vi "Control Experiment.vi"(8 "Error In":errorcluster, 9 "KH":T5={"KH #"=[0, 1, 2, 3, 4, 5, 6, 7, 8, 9, 10, 11, 12, 13, 14, 15], "KH Configuration"=[enum."SE+ (-gnd)", enum."SE+ (-gnd)", enum."Differential", enum."Differential", enum."SE+ (-gnd)", enum."Differential", enum."Differential", enum."SE+ (-gnd)", enum."Differential", enum."Differential", enum."SE+ (-gnd)", enum."SE+ (-gnd)", enum."Differential", enum."Ground", enum."Ground", enum."Ground"], "KH Gain"=[enum."1000x", enum."1000x", enum."1000x", enum."1000x", enum."1000x", enum."1000x", enum."1000x", enum."1000x", enum."1000x", enum."1000x", enum."1000x", enum."1000x", enum."1000x", enum."1000x", enum."1000x", enum."100x"], "KH Shunt Resistor"=[enum."Open", enum."Open", enum."Open", enum."5k Ohms", enum."Open", enum."Open", enum."5k Ohms", enum."Open", enum."Open", enum."5k Ohms", enum."Open", enum."Open", enum."50k Ohms", enum."Open", enum."Open", enum."Open"]}, 10 "Lockin":T7={"AI"=[1, 2, 3, 4, 5, 6, 7, 8, 9, 10, 11, 12, 13, 14, 15, 16], "Electrode"=["4", "5", "6", "7", "9", "11", "12", "13", "16", "17", "20", "21", "1", "", "", ""], "Label"=[12, 14, 15, 13, 10, 11, 9, 8, 4, 2, 1, 3, 6, 0, 0, 0], "Electrode Config"=[enum."Current", enum."Voltage (SE)", enum."Voltage (SE)", enum."Current", enum."Voltage (SE)", enum."Voltage (SE)", enum."Current", enum."Current", enum."Voltage (SE)", enum."Current", enum."Current", enum."Voltage (SE)", enum."Gate", enum."Voltage (SE)", enum."Voltage (SE)", enum."Voltage (SE)"]} {"Label" items=["", "I+", "I-", "V1+", "V1-", "dV1", "Vsg", "Vbg", "I2+", "I2-", "V2+", "V2-", "I3+", "I3-", "V3+", "V3-"]}) -> (0 "Error Out":errorcluster)   [LabVIEW 2019, in "Control Experiment.lvclass"]
doc: "Use this VI to help configure your experiment.\n1. Choose Pickering or Not Pickering\n2. Configure the Electrode control to show which electrode is connected to which lockin\n3. Choose a Label for each electrode to configure Krohn Hite amplifier automatically\n4. Easily set all Krohn Hite channels to be \"all ground\" or \"all differential\" mode\n5. Fill out information about you and your device in the lower left corner\n6. When you are finished, or when you want to update the amplifiers, click the \"CREATE OUTPUT\" button located in upper right. Clicking this button will set the amplifiers, Pickering switch (if you have one), and write information to a functional global variable that you can easily read from elsewhere in your program"
uses:
  Control Experiment.lvclass
  Typedefs/Instrument--enum.ctl
  <userlib>/LevyLab/Krohn Hite 7008/typedefs/Shunt-Enum.ctl
  Typedefs/KH Mode-enum.ctl
  <userlib>/LevyLab/Krohn Hite 7008/typedefs/Input Configuration-Enum.ctl
  <userlib>/LevyLab/Krohn Hite 7008/typedefs/Gain-Enum.ctl
  <userlib>/LevyLab/Krohn Hite 7008/typedefs/SetAll-Array.ctl
  <userlib>/LevyLab/Krohn Hite 7008/typedefs/SetAll-Cluster.ctl
  <userlib>/LevyLab/Krohn Hite 7008/typedefs/Channel-Enum.ctl
  <userlib>/LevyLab/Krohn Hite 7008/typedefs/Filter-Enum.ctl
  <userlib>/LevyLab/Krohn Hite 7008/typedefs/Coupling-Enum.ctl
  <userlib>/LevyLab/Instrument Framework/SMOs/Configuration/Configuration.lvclass
  Typedefs/UI Controls --cluster.ctl
  <userlib>/LevyLab/Instrument Framework/SMOs/Logger.PGSQL/Logger.PGSQL.lvclass
  C:/Program Files (x86)/National Instruments/LabVIEW 2019/vi.lib/JKI/JKI SMO/SMO/SMO.lvclass
  Control Experiment.lvclass/Control Experiment.ctl
  <userlib>/_MGI/File/MGI Create Directory Chain Behavior Enum.ctl
  Typedefs/Control Experiment JSON--cluster.ctl
  <userlib>/LevyLab/Krohn Hite 7008/Instrument.KH7008.lvclass/Instrument.KH7008.ctl
  23189d07-d529-447d-957d-13a42bf56e57.vi
  9a447b37-f4f5-4836-8e27-fdda23b4a061.vi
  <vilib>/JDP Science/JSONtext/Variant to JSON Text.vi
  <vilib>/regexp/Match Regular Expression.xnode
  <vilib>/JDP Science/JSONtext/LVClass Serializer/JSONtext LVClass Serializer.lvclass
  <userlib>/LevyLab/Krohn Hite 7008/Instrument.KH7008.lvclass
  <vilib>/JKI/JKI SMO/SMO/SMO.lvclass
  <userlib>/LevyLab/Lockin-Multichannel/Instrument.Lockin/Instrument.Lockin.lvclass
  C:/Program Files (x86)/National Instruments/LabVIEW 2019/user.lib/LevyLab/Instrument Framework/SMOs/Logger/Logger.lvclass
panel:
  out "KH Addresses":refnum<visa-resource-name>[](array[refnum])=["COM20", "COM14"] caption="KH Address[A,B,C,...]"
  in  "I'm Finished Taking Data!":bool
  out "Values have changed":bool=TRUE
  in  "Create Output":bool
  in  "OK":bool
  out "Control Experiment":refnum<class "Control Experiment.lvclass">
  in  "C.E.":refnum<class "Control Experiment.lvclass">
  in  "Tab Control":T1(tab)
  out "state":string="    devices:\n    \n    1. 80x80um rectangle\n    2. hash: 200 horizontal and vertical lines 400nm apart\n    3. hash structures: 400, 200nm apart horizontal and vertical lines"
  in  "Instrument Configuration":bool
  out "Instruments":string="    devices:\n    \n    1. 80x80um rectangle\n    2. hash: 200 horizontal and vertical lines 400nm apart\n    3. hash structures: 400, 200nm apart horizontal and vertical lines"
  in  "DC Coupled":bool=TRUE
  in  "Bandwidth Filter":bool=TRUE
  in  "AO Channels":u32=8
  in  "Gain":dbl[](array[numeric])=[1.0, 1.0, 1.0, 1.0, 1.0, 1.0, 1.0, 1.0, 1.0, 1.0, 1.0, 1.0, 1.0, 1.0, 1.0, 1.0]
  in  "AI Channels":u32=16
  in  "KH All Buttons":T8(radio)
  in  "Defualt Shunt Resistor":T4=enum."5k Ohms"
  in  "Description":string="    devices:\n    \n    1. 80x80um rectangle\n    2. hash: 200 horizontal and vertical lines 400nm apart\n    3. hash structures: 400, 200nm apart horizontal and vertical lines"
  in  "Sample (SAXXXX)":string="SA40178"
  in  "Device (YYYYMMDD)":string="20210125"
  in  "Instrument":T9=enum."MNK"
  in  "Username":string="Aditi"
  in  "non KH":T10 {"Labels 2" items=["", "I+", "I-", "V1+", "V1-", "dV1", "Vsg", "Vbg", "I2+", "I2-", "V2+", "V2-", "I3+", "I3-", "V3+", "V3-"]}
  in  "Ring":u16(ring)=2 items=["----Sweep Control----", "Sweep Control.vi", "Continuous B Sweep.vi", "----Transport----", "IV.vi", "IV_Sweep.vi", "Lockin_time.vi", "Lockin_Vsg.vi", "Lockin_sweep.vi", "Lockin_AIWFM_time.vi", "THz_TimeDelay.vi", "Sweep_AIWFM_time.vi"]
  in  "Open VI":bool
  in  "Open Lockin":bool
  in  "Default Path":path=path "C:/temp" caption="Default Path (Do not add your instrument name here)(Typ. G:\\My Drive\\ansom\\Data)"
  out "Comments":string="Device: \r  Device Name: SA40178.20210125\r  Computer: KHOLEK\r  User: Aditi\r  Instrument: MNK\r  Description: |\r        devices:\r        \r        1. 80x80um rectangle\r        2. hash: 200 horizontal and vertical lines 400nm apart\r        3. hash structures: 400, 200nm apart horizontal and vertical lines\r\rExperiment: \r  Time: 2021-02-22T11:02:02\r  Description: |\r\rSweep: \r- Loop1: [OFF, 0.000000]\r- Loop2: [OFF, 0.000000]\r- Loop3: [OFF, 0.000000]\r- Loop4: [OFF, 0.000000]\r\rWiring: \r- Electrode 4: Lockin 1, V2, KH1 Channel 1, SE+ (-gnd), 1000x, Open\r- Electrode 5: Lockin 2, V2, KH1 Channel 2, SE+ (-gnd), 1000x, Open\r- Electrode 6: Lockin 3, I2, KH1 Channel 3, Differential, 1000x, 5k Ohms\r- Electrode 7: Lockin 4, I2, KH1 Channel 4, Differential, 1000x, 5k Ohms\r- Electrode 9: Lockin 5, V2, KH1 Channel 5, SE+ (-gnd), 1000x, Open\r- Electrode 11: Lockin 6, I2, KH1 Channel 6, Differential, 1000x, 5k Ohms\r- Electrode 12: Lockin 7, I2, KH1 Channel 7, Differential, 1000x, 5k Ohms\r- Electrode 13: Lockin 8, V2, KH1 Channel 8, SE+ (-gnd), 1000x, Open\r- Electrode 16: Lockin 9, I-, KH2 Channel 1, Differential, 1000x, 5k Ohms\r- Electrode 17: Lockin 10, I+, KH2 Channel 2, Differential, 1000x, 5k Ohms\r- Electrode 20: Lockin 11, V1+, KH2 Channel 3, SE+ (-gnd), 1000x, Open\r- Electrode 21: Lockin 12, V1-, KH2 Channel 4, SE+ (-gnd), 1000x, Open\r- Electrode 1: Lockin 13, Vsg, KH2 Channel 5, Differential, 1000x, 50k Ohms\r\rLockin: \r  AO: \r  - AO 1: amp = 0.000 mV, DC = 0.000 mV, f = 1.00 Hz, phi = 0.00°, Triangle\r  - AO 2: amp = 0.000 mV, DC = 0.000 mV, f = 1.00 Hz, phi = 0.00°, Triangle\r  - AO 3: amp = 0.000 mV, DC = 0.000 mV, f = 1.00 Hz, phi = 0.00°, Triangle\r  - AO 4: amp = 0.000 mV, DC = 0.000 mV, f = 1.00 Hz, phi = 0.00°, Triangle\r  - AO 5: amp = 0.000 mV, DC = 0.000 mV, f = 1.00 Hz, phi = 0.00°, Triangle\r  - AO 6: amp = 10.000 mV, DC = 0.000 mV, f = 1.00 Hz, phi = 0.00°, Triangle\r  - AO 7: amp = 0.000 mV, DC = 0.000 mV, f = 1.00 Hz, phi = 0.00°, Triangle\r  - AO 8: amp = 0.000 mV, DC = 0.000 mV, f = 1.00 Hz, phi = 0.00°, Triangle\r  - AO 9: amp = 0.000 mV, DC = 0.000 mV, f = 1.00 Hz, phi = 0.00°, Triangle\r  - AO 10: amp = 10.000 mV, DC = 0.000 mV, f = 1.00 Hz, phi = 0.00°, Triangle\r  - AO 11: amp = 0.000 mV, DC = 0.000 mV, f = 1.00 Hz, phi = 0.00°, Triangle\r  - AO 12: amp = 0.000 mV, DC = 0.000 mV, f = 1.00 Hz, phi = 0.00°, Triangle\r  - AO 13: amp = 0.000 mV, DC = 0.000 mV, f = 1.00 Hz, phi = 0.00°, Sine\r  - AO 14: amp = 0.000 mV, DC = 0.000 mV, f = 1.00 Hz, phi = 0.00°, Sine\r  - AO 15: amp = 0.000 mV, DC = 0.000 mV, f = 1.00 Hz, phi = 0.00°, Sine\r  - AO 16: amp = 0.000 mV, DC = 0.000 mV, f = 1.00 Hz, phi = 0.00°, Sine\r  - AO 17: amp = 0.000 mV, DC = -0.000 mV, f = 1.00 Hz, phi = 0.00°, Sine\r  - AO 18: amp = 0.000 mV, DC = 0.000 mV, f = 1.00 Hz, phi = 0.00°, Sine\r  - AO 19: amp = 0.000 mV, DC = 0.000 mV, f = 1.00 Hz, phi = 0.00°, Sine\r  - AO 20: amp = 0.000 mV, DC = 0.000 mV, f = 1.00 Hz, phi = 0.00°, Sine\r  - AO 21: amp = 0.000 mV, DC = 0.000 mV, f = 1.00 Hz, phi = 0.00°, Sine\r  - AO 22: amp = 0.000 mV, DC = 0.000 mV, f = 1.00 Hz, phi = 0.00°, Sine\r  - AO 23: amp = 0.000 mV, DC = 0.000 mV, f = 1.00 Hz, phi = 0.00°, Sine\r  - AO 24: amp = 0.000 mV, DC = 0.000 mV, f = 1.00 Hz, phi = 0.00°, Sine\r  REF: \r  - Lockin 1: f = 1.00 Hz, phi = 0.00°, TC = 0.10 s, order = 2 \r  Sampling: \r  - Fs: 10000.000000\r  - N: 1000\r"
  out "Device Folder":path=path "D:/Data/MNK/SA40178.20210125" caption="(\\base path\\project\\device\\ )"
  out "JSON String":string="{\r\n    \"Device\":{\r\n        \"Device\":\"SA40178.20210125\",\r\n        \"User\":\"Aditi\",\r\n        \"Time\":\"2021-02-22T11:02:02\",\r\n        \"Computer Name\":\"KHOLEK\"\r\n    },\r\n    \"Wiring\":{\r\n        \"Lockin Ch\":[\r\n            1,\r\n            2,\r\n            3,\r\n            4,\r\n            5,\r\n            6,\r\n            7,\r\n            8,\r\n            9,\r\n            10,\r\n            11,\r\n            12,\r\n            13,\r\n            14,\r\n            15,\r\n            16\r\n        ],\r\n        \"KH Electrodes\":[\r\n            \"4\",\r\n            \"5\",\r\n            \"6\",\r\n            \"7\",\r\n            \"9\",\r\n            \"11\",\r\n            \"12\",\r\n            \"13\",\r\n            \"16\",\r\n            \"17\",\r\n            \"20\",\r\n            \"21\",\r\n            \"1\",\r\n            \"\",\r\n            \"\",\r\n            \"\"\r\n        ],\r\n        \"KH Labels\":[\r\n            \"V2\",\r\n            \"V2\",\r\n            \"I2\",\r\n            \"I2\",\r\n            \"V2\",\r\n            \"I2\",\r\n            \"I2\",\r\n            \"V2\",\r\n            \"I-\",\r\n            \"I+\",\r\n            \"V1+\",\r\n            \"V1-\",\r\n            \"Vsg\",\r\n            \"\",\r\n            \"\",\r\n            \"\"\r\n        ],\r\n        \"Other Electrodes\":[\r\n            \"4\",\r\n            \"5\",\r\n            \"6\",\r\n            \"7\",\r\n            \"9\",\r\n            \"11\",\r\n            \"12\",\r\n            \"13\",\r\n            \"16\",\r\n            \"17\",\r\n            \"20\",\r\n            \"21\",\r\n            \"1\",\r\n            \"\",\r\n            \"\",\r\n            \"\"\r\n        ],\r\n        \"Other Labels\":[\r\n            \"V2\",\r\n            \"V2\",\r\n            \"I2\",\r\n            \"I2\",\r\n            \"V2\",\r\n            \"I2\",\r\n            \"I2\",\r\n            \"V2\",\r\n            \"I-\",\r\n            \"I+\",\r\n            \"V1+\",\r\n            \"V1-\",\r\n            \"Vsg\",\r\n            \"\",\r\n            \"\",\r\n            \"\"\r\n        ]\r\n    }\r\n}"
  in  "Labels Strings":string[](array[string])=["", "I+", "I-", "V1+", "V1-", "dV1", "Vsg", "Vbg", "I2+", "I2-", "V2+", "V2-", "I3+", "I3-", "V3+", "V3-"]
  out "YAML example":string="description: This is a dummy dataset which mimics smFRET data.\n\nsetup:\n    ## Mandatory fields\n    num_pixels: 2                # using 2 detectors\n    num_spots: 1                 # a single confocal excitation\n    num_spectral_ch: 2           # donor and acceptor detection\n    num_polarization_ch: 1       # no polarization selection\n    num_split_ch: 1              # no beam splitter\n    modulated_excitation: False  # CW excitation, no modulation\n    lifetime: False              # no TCSPC in detection\n\n    ## Optional fields\n    excitation_wavelengths:      # List of excitation wavelenghts\n       - !!float 532e-9\n    excitation_cw:               # List of booleans, True if wavelength is CW\n       - True\n    detection_wavelengths:       # Nominal center wavelength for each for detection ch\n       - !!float 580e-9\n       - !!float 640e-9\n\nsample:\n  sample_name: describe the sample here\n  buffer_name: describe the buffer here\n  dye_names: 'Cy3B, ATTO647N'   # Comma separates names of fluorophores\n\nidentity:\n    author: Author Name\n    author_affiliation: Name of Research Institution\n\nprovenance:\n    filename: 'photon_data.hdf5'\n    software: Acquisition Software Name\n\nphoton_data:\n    timestamps_specs:\n        timestamps_unit: !!float 10e-9  # 10 ns\n    measurement_specs:\n        measurement_type: smFRET\n        detectors_specs:\n            spectral_ch1: [0]  # list of donor's detector IDs\n            spectral_ch2: [1]  # list of acceptor's detector IDs"
  in  "String":string
  # "SANDBOX:"
  # "Sample"
  # "Krohn Hite"
  # "Lockin"
  # "Lockin"
  # "Krohn Hite"
  # "Other"
  # "Device and Project Description"
  # "Instrument Configuration"
  # "Experiment VIs"
  # "Path Configuration"
  # "Use this VI to help configure your experiment.\n1. Configure the Electrode control to show which electrode is connected to which lockin\n2. Choose a Label for each electrode to configure Krohn Hite amplifier automatically\n3. Easily set all Krohn Hite channels to be \"all ground\" or \"all differential\" mode\n4. Fill out information about you and your device in the lower left corner\n5. When you are finished, or when you want to update the amplifiers, click the \"CREATE OUTPUT\" button located in upper right.\nClicking this button will set the amplifiers, Pickering switch (if you have one), and write information to a functional global variable that you can easily read from elsewhere in your program"
  # "If you want to have new labels for the \"Labels\" field you can type them here"
  # "The magic words are:\nI\nVsg\nVbg\nVtg\ndV\nV"
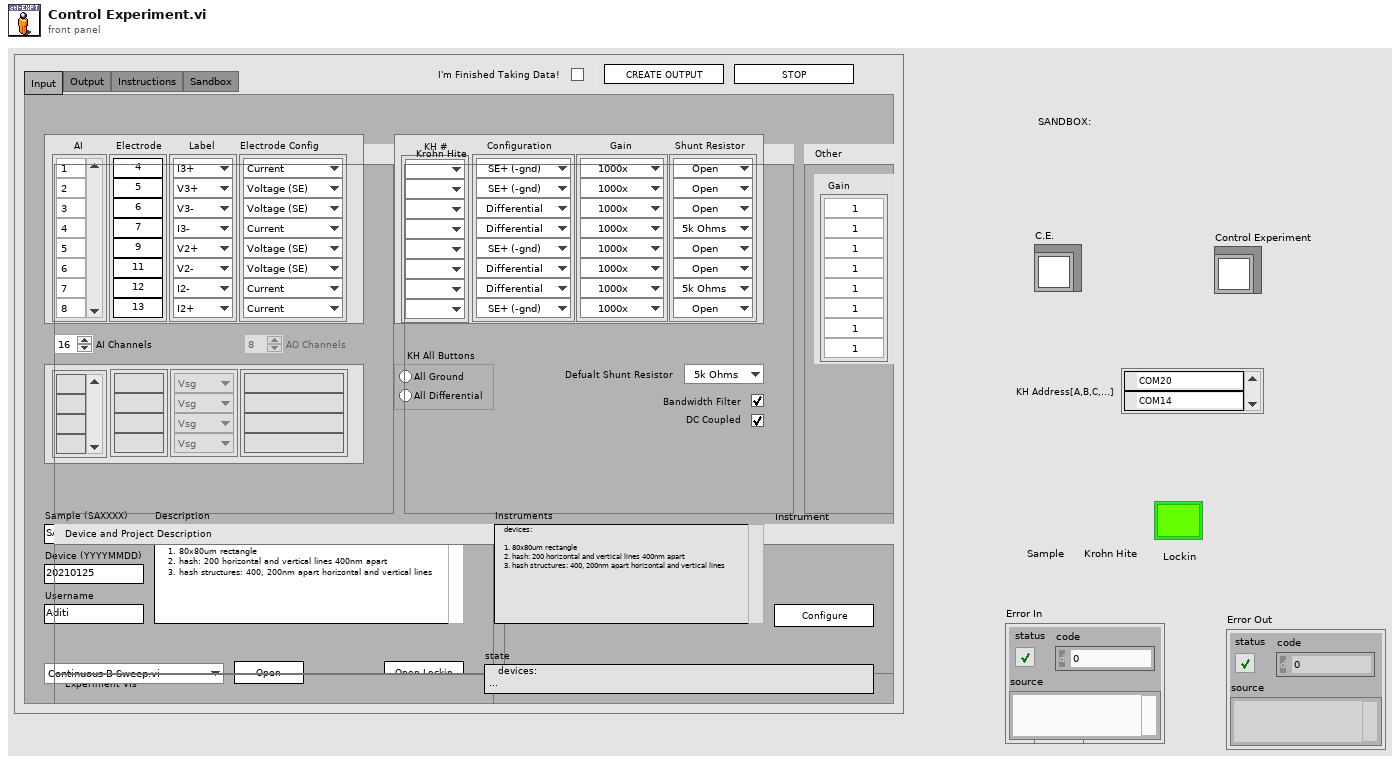
[diagram p1: front panel]
types:
  T1 = enum32{"Input", "Output", "Instructions", "Sandbox"}
  T2 = typedef "Instrument.KH7008.lvclass/Input Configuration-Enum.ctl" = enum16{"Ground", "SE+ (-gnd)", "SE- (+gnd)", "Differential"}
  T3 = typedef "Instrument.KH7008.lvclass/Gain-Enum.ctl" = enum16{"1x", "10x", "100x", "1000x"}
  T4 = typedef "Instrument.KH7008.lvclass/Shunt-Enum.ctl" = enum16{"Open", "50 Ohms", "500 Ohms", "5k Ohms", "50k Ohms", "10M Ohm"}
  T5 = cluster{"KH #":u16[], "KH Configuration":T2[], "KH Gain":T3[], "KH Shunt Resistor":T4[]}
  T6 = typedef "Control Experiment.lvclass/KH Mode-enum.ctl" = enum16{"Ground", "Current", "Voltage (SE)", "Voltage (Diff)", "Gate"}
  T7 = cluster{"AI":u32[], "Electrode":string[], "Label":u16[], "Electrode Config":T6[]}
  T8 = enum32{"No Selection", "All Ground", "All Differential"}
  T9 = typedef "Control Experiment.lvclass/Instrument--enum.ctl" = enum16{"----- AFM/EBL -----", "AGILENT", "CYPHER", "Gemini2", "JEOL", "MFP3D", "----- Cryostat -----", "CF900", "DR200", "MNK", "PPMS (simulated)", "PPMS 1", "PPMS 2", "PPMS 3", "----- Optics -----", "THz 1 (Element 2/Montana)", "THz 2 (Tsunami/Janis)"}
  T10 = cluster{"Scroll Bar":string[], "Electrodes 2":string[], "Labels 2":u16[], "unused":string[]}
  T11 = enum32{"invalid app kind", "Development System", "Run Time System", "Student Edition", "Embedded LabVIEW", "Evaluation", "Custom"}
  T12 = enum32{"Bad", "Idle", "Run top level", "Running"}
  T13 = enum32{"Invalid", "Standard", "Closed", "Hidden", "Minimized", "Maximized"}
  T14 = typedef "MGI Create Directory Chain Behavior Enum.ctl" = enum16{"Auto Detect", "Path Contains a File", "Path Does Not Contain a File"}
  T15 = typedef "Instrument.KH7008.lvclass/SetAll-Cluster.ctl" = cluster{"Channel":T16, "Gain":T3, "Bandwidth Filter":T17, "Shunt Resistor":T4, "Coupling":T18, "Input Config":T2}
  T16 = typedef "Instrument.KH7008.lvclass/Channel-Enum.ctl" = enum16{"Channel 1", "Channel 2", "Channel 3", "Channel 4", "Channel 5", "Channel 6", "Channel 7", "Channel 8"}
  T17 = typedef "Instrument.KH7008.lvclass/Filter-Enum.ctl" = enum16{"OFF", "ON"}
  T18 = typedef "Instrument.KH7008.lvclass/Coupling-Enum.ctl" = enum16{"AC", "DC"}
  T19 = typedef "Control Experiment.lvclass/Experiment Description--cluster.ctl" = cluster{"User":string, "Device":string, "Device Path":path, "Device Description":string, "Experiment Path":path, "Experiment Description":string, "Instrument":T9, "Instruments":cluster{"class path":path, "Address":string, "Type":T20}[], "Sweep":cluster{"key":string, "value":variant}[]}
  T20 = typedef "Control Experiment.lvclass/Instrument Types--combo.ctl" = string
  T21 = typedef "Control Experiment.lvclass/Wiring Description--cluster.ctl" = cluster{"Lockin Ch":i32[], "KH":cluster{"Electrodes":string[], "Labels":string[]}, "not KH":cluster{"Electrodes":string[], "Labels":string[]}}
  T22 = typedef "Instrument.KH7008.lvclass/SetAll-Array.ctl" = T15[]
  T23 = typedef "Control Experiment.lvclass/UI Controls --cluster.ctl" = cluster{"Sample":string, "Device":string, "Username":string, "Description":string, "Default Path":path, "AWS Path":path, "Instrument":T9, "Lockin?":bool, "Lockin Address":string, "Krohn Hite?":bool, "KH Addresses":refnum<visa-resource-name>[], "KH All Buttons":enum32{"No Selection", "All Ground", "All Differential"}, "Strain Cell?":bool, "Strain Cell Address":refnum<visa-resource-name>, "C Bridge?":bool, "Capacitance Bridge Address":refnum<visa-resource-name>, "Lockin":cluster{"AI":u32[], "Electrode":string[], "Label":u16[], "Electrode Config":T6[]}, "KH":cluster{"KH #":enum16{"A 1", "A 2", "A 3", "A 4", "A 5", "A 6", "A 7", "A 8", "B 1", "B 2", "B 3", "B 4", "B 5", "B 6", "B 7", "B 8", "none"}[], "KH Configuration":T2[], "KH Gain":T3[], "KH Shunt Resistor":T4[], "Filter":bool, "DC Coupled":bool}, "non KH":cluster{"Scroll Bar":string[], "Electrodes 2":string[], "Labels 2":u16[], "unused":string[]}}
  T24 = cluster{"Core":cluster{"Current VI Reference":refnum<vi>, "Close Panel on Exit?":bool}, "C.E.":refnum<class "Control Experiment.lvclass">, "Experiment":T19, "Wiring Configuration":T21, "Channel Settings":cluster{"Channel Setting":T22}[], "KH All Buttons":enum32{"No Selection", "All Ground", "All Differential"}, "Lockin":cluster{"AI":u32[], "Electrode":string[], "Label":u16[], "Electrode Config":T6[]}, "KH":cluster{"KH #":u16[], "KH Configuration":T2[], "KH Gain":T3[], "KH Shunt Resistor":T4[]}, "non KH":cluster{"Scroll Bar":string[], "Electrodes 2":string[], "Labels 2":u16[], "unused":string[]}, "UI":T23, "Logger":refnum<class "Logger.PGSQL.lvclass">, "Config":refnum<class "Configuration.lvclass">, "VI paths":path[], "top level?":bool}
  T25 = cluster{"Current VI Reference":refnum<vi>, "Close Panel on Exit?":bool}
  T26 = enum16{"A 1", "A 2", "A 3", "A 4", "A 5", "A 6", "A 7", "A 8", "B 1", "B 2", "B 3", "B 4", "B 5", "B 6", "B 7", "B 8", "none"}[]
  T27 = cluster{"class path":path, "Address":string, "Type":T20}[]
  T28 = typedef "Control Experiment.lvclass/Control Experiment JSON--cluster.ctl" = cluster{"Device":cluster{"Device":string, "User":string, "Time":string, "Computer Name":string}, "Wiring":cluster{"Lockin Ch":u32[], "KH Electrodes":string[], "KH Labels":string[], "Other Electrodes":string[], "Other Labels":string[]}}
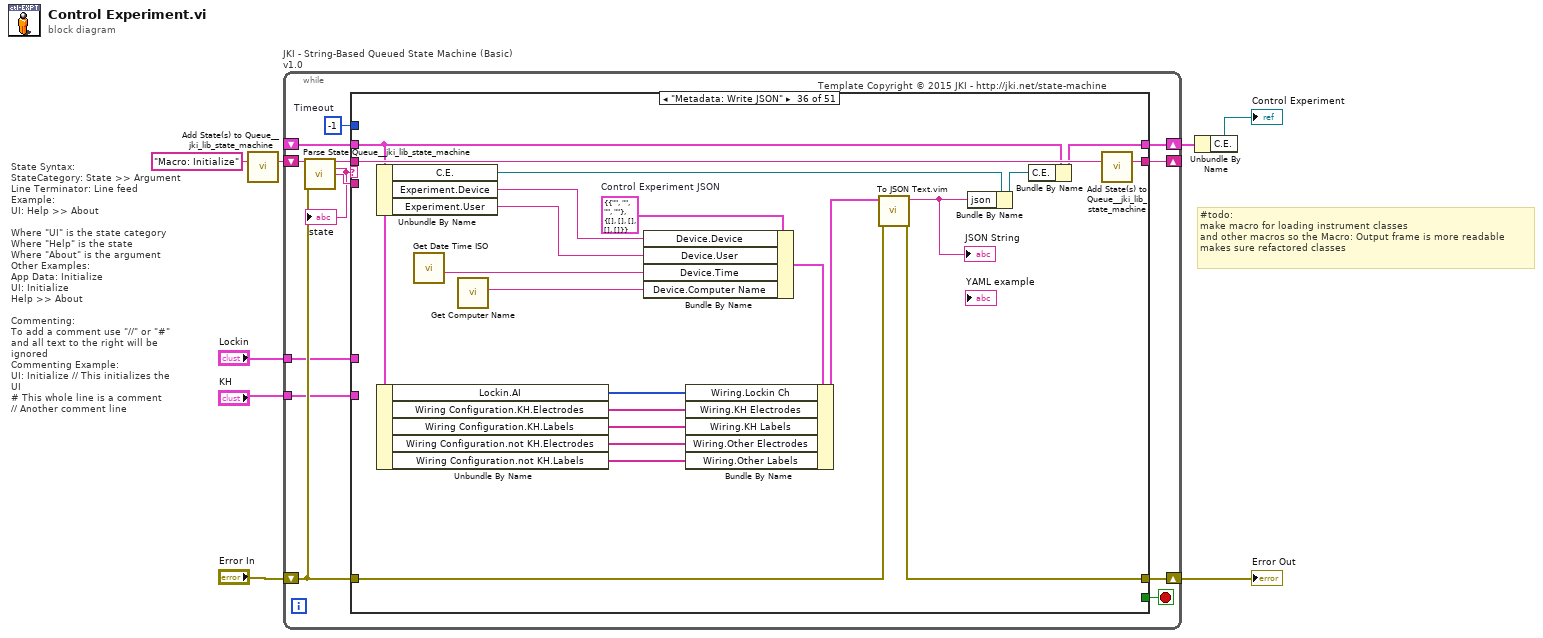
[diagram p0: block diagram]
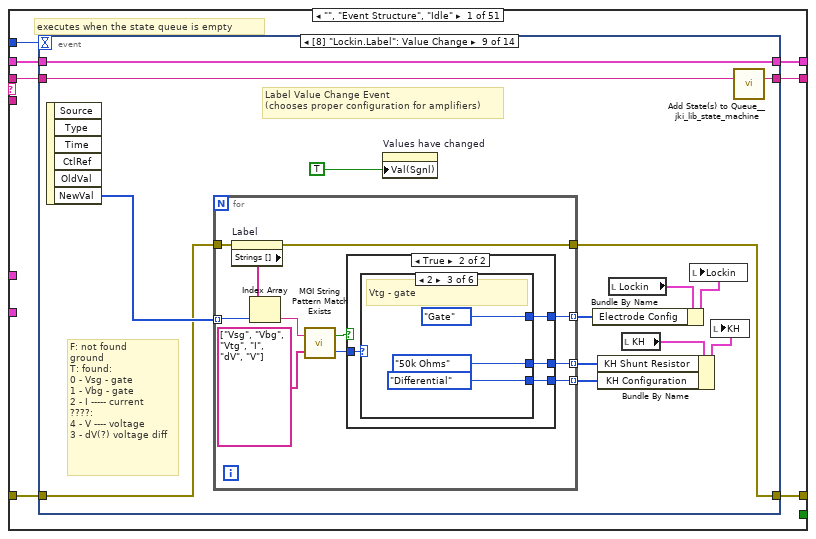
[diagram p2: hidden frame]
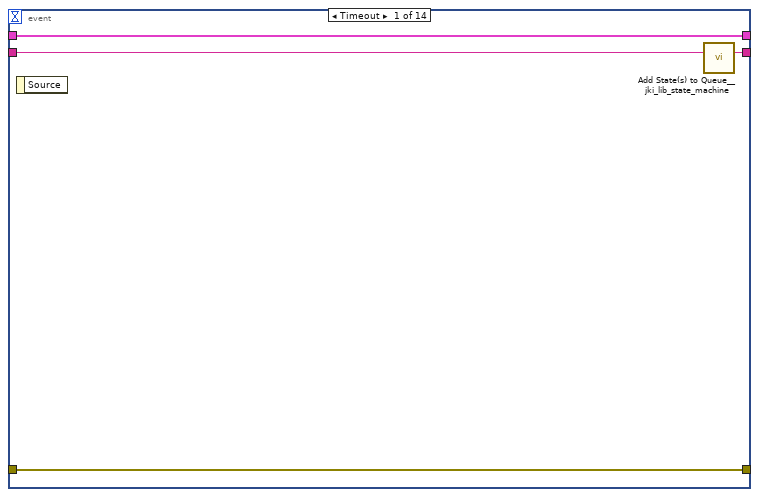
[diagram p3: hidden frame]
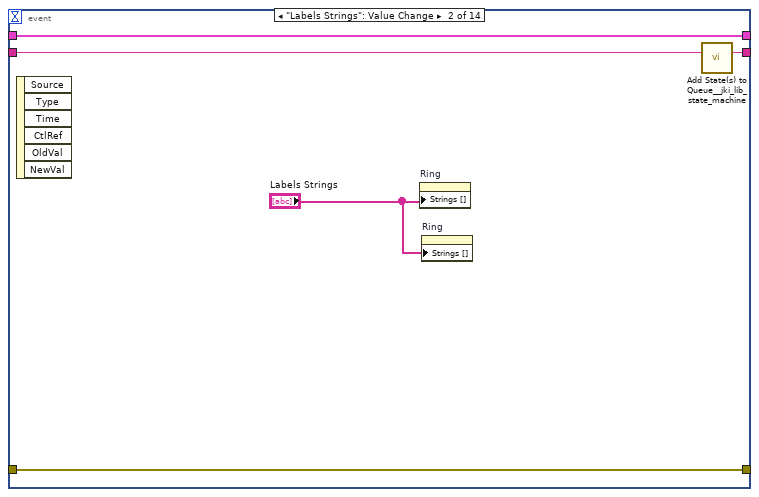
[diagram p4: hidden frame]
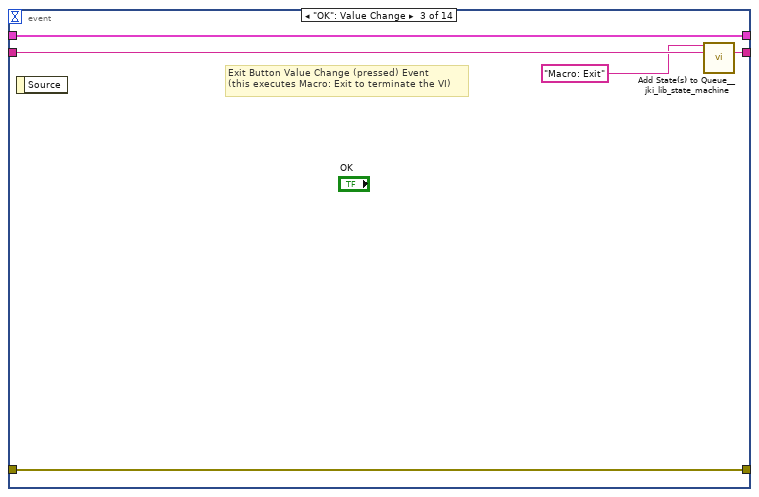
[diagram p5: hidden frame]
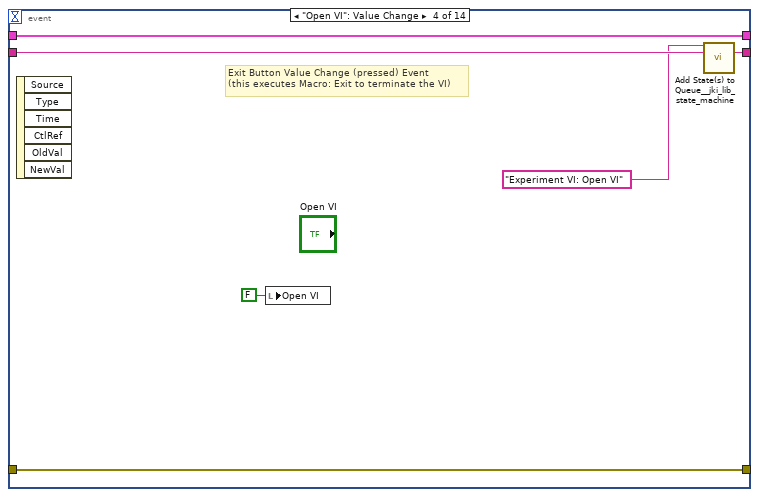
[diagram p6: hidden frame]
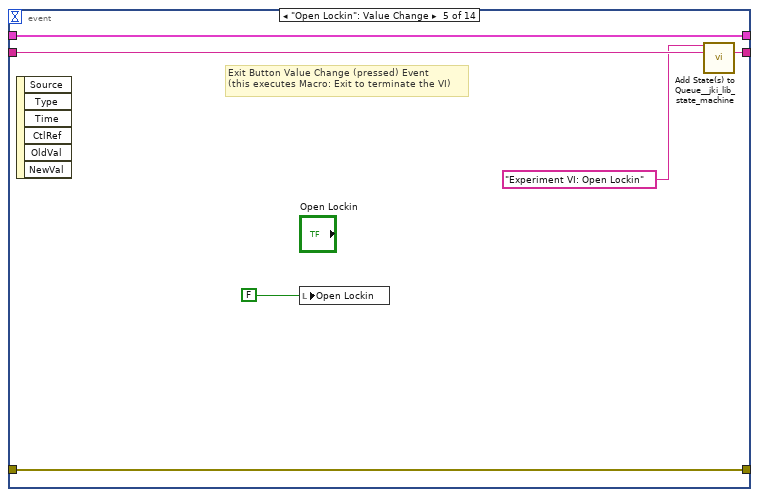
[diagram p7: hidden frame]
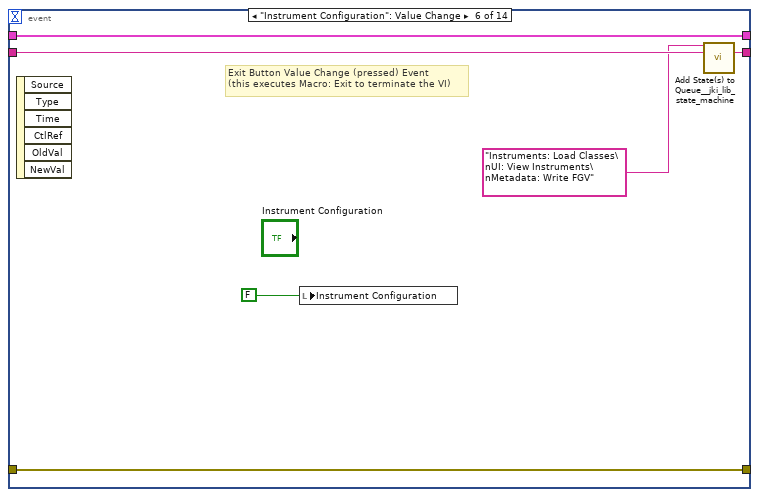
[diagram p8: hidden frame]
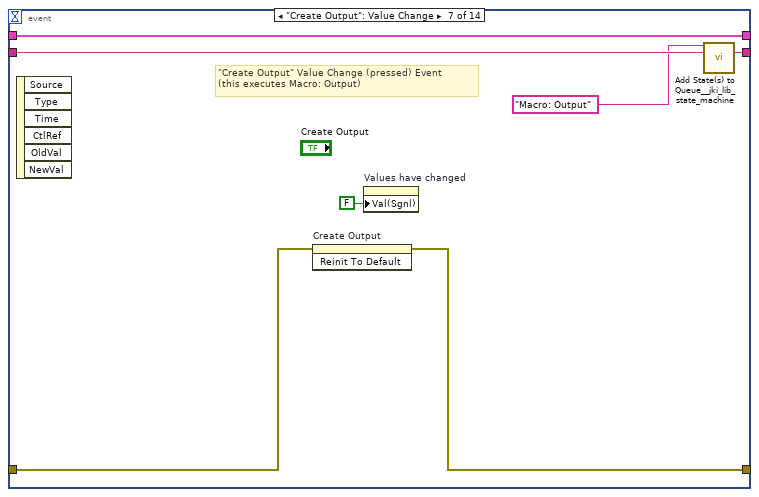
[diagram p9: hidden frame]
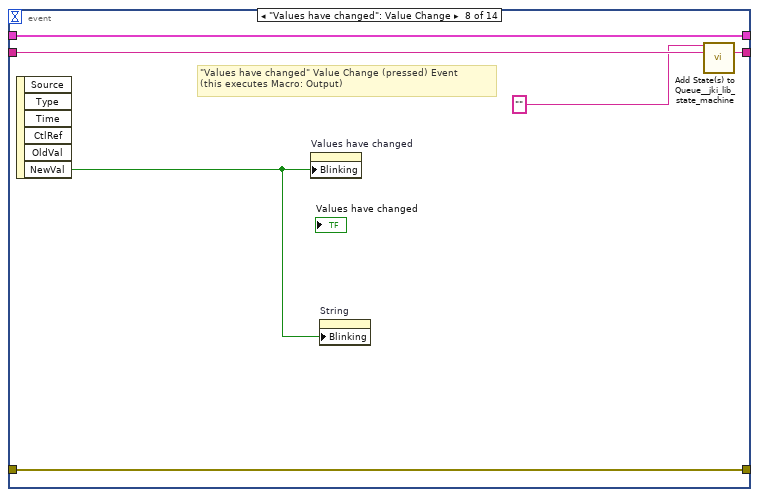
[diagram p10: hidden frame]
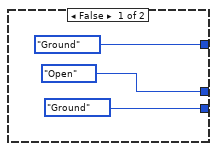
[diagram p11: hidden frame]
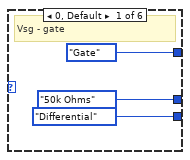
[diagram p12: hidden frame]
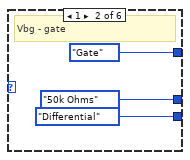
[diagram p13: hidden frame]
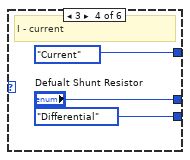
[diagram p14: hidden frame]
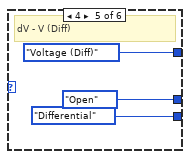
[diagram p15: hidden frame]
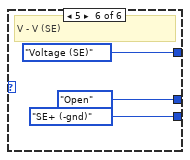
[diagram p16: hidden frame]
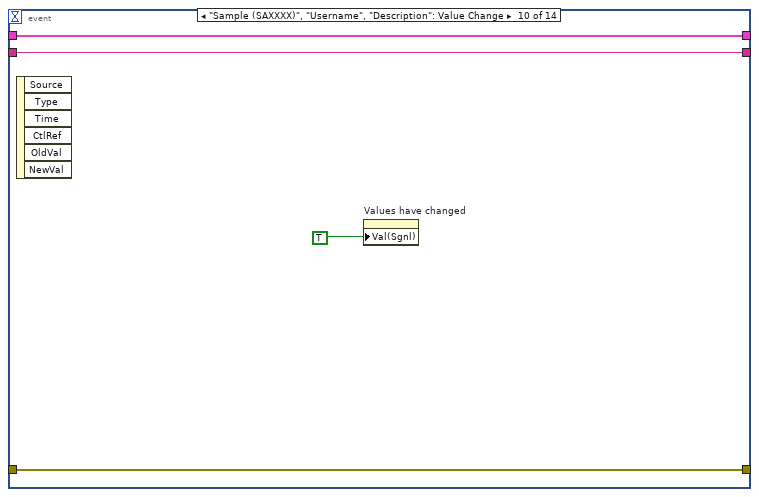
[diagram p17: hidden frame]
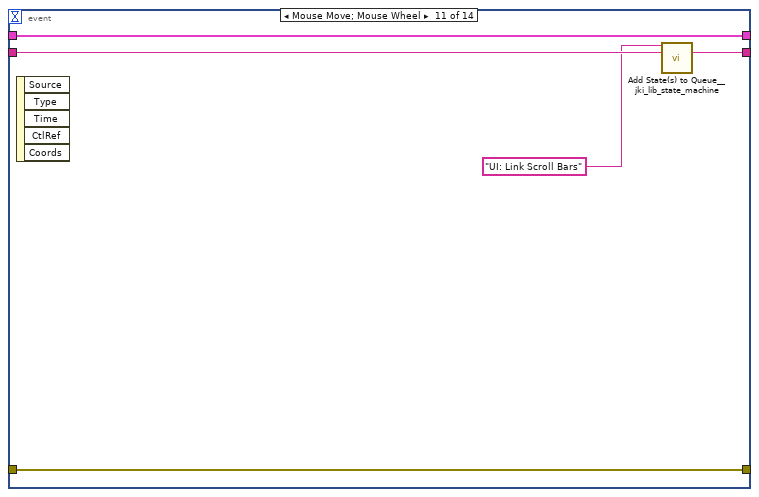
[diagram p18: hidden frame]
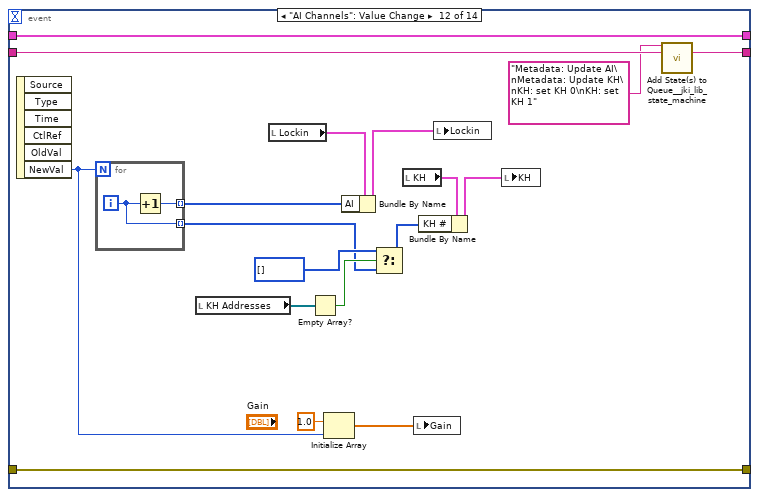
[diagram p19: hidden frame]
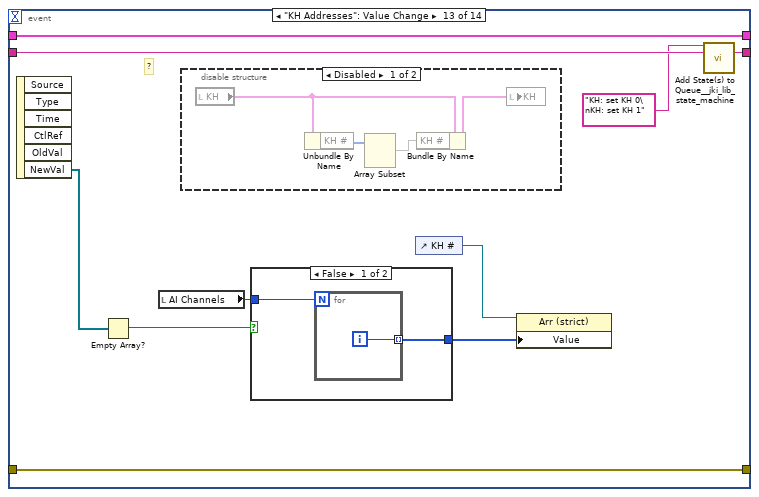
[diagram p20: hidden frame]
diagram:
  # "#todo:\nmake macro for loading instrument classes\nand other macros so the Macro: Output frame is more readable\nmakes sure refactored classes"
  # "State Syntax:\nStateCategory: State >> Argument\nLine Terminator: Line feed\nExample:\nUI: Help >> About\n\nWhere \"UI\" is the state category\nWhere \"Help\" is the state\nWhere \"About\" is the argument\nOther Examples:\nApp Data: Initialize\nUI: Initialize\nHelp >> About\n\nCommenting:\nTo add a comment use \"//\" or \"#\" and all text to the right will be ignored\nCommenting Example:\nUI: Initialize // This initializes the UI\n# This whole line is a comment\n// Another comment line"
  n1 = call <vilib>:"Add State(s) to Queue__jki_lib_state_machine.vi"("State(s) in (\"\")"="Macro: Initialize") -> ("States Out"=w8:string)  [unwired: 14 in]
  n2 = while "JKI - String-Based Queued State Machine (Basic) v1.0" {
    shift-right: [w15] -> w6
    shift-left: _ -> [w14]
    shift-right: [w18] -> w2
    shift-left: "Error In" -> [w12]
    shift-right: [w17] -> _
    shift-left: w8 -> [w19]
    tunnel: "Lockin" -> [w11]
    tunnel: "KH" -> [w10]
    stop <- w16 stop-if-true
    w13 = -1  # Timeout
    # "Template Copyright © 2015 JKI - http://jki.net/state-machine"
    n3 = call <vilib>:"Parse State Queue__jki_lib_state_machine.vi"("State Queue"=w19, "Error In (no error)"=w12) -> ("Remaining States"=w21:string, "Current State"=w9:string, "Arguments"=w20:string)  [unwired: 11 in]
    "state" <- w9
    n4 = case shown="\"Metadata: Write JSON\"" w9 {
      selector: w9 -> [_ _ w181 _ _ _ _ _ _ _ _ _ _ _ _ _ _ _ _ _ _ _ _ _ _ _ _ _ _ _ _ _ _ _ _ _ _ _ _ _ _ _ _ _ _ _ _ _ _ _ _]
      tunnel: w21 -> [w28 w180 w185 w203 w209 w214 w218 w236 w247 w262 w288 w298 w302 w315 w340 w352 w365 w376 w402 w417 w430 w434 w439 w450 w457 w470 w475 w479 w491 w507 w531 w590 w649 w772 w785 w806 w813 w821 w825 w842 w881 w968 w983 w993 w1007 w1028 w1042 w1047 w1051 w1061 w1079]
      tunnel: w20 -> [_ _ _ _ _ _ _ _ _ _ _ _ _ _ _ _ w360 w370 _ _ _ _ _ _ _ _ _ _ _ _ _ _ _ _ _ _ _ _ _ _ _ _ _ _ _ _ _ _ _ _ _]
      tunnel: w14 -> [w26 w177 w183 w194 w206 w212 w215 _ w242 w258 w273 w293 w299 w305 w318 w349 w363 w372 w399 w414 w428 w431 w436 w447 w455 w467 w472 w476 w487 w503 w529 w588 w647 w768 w783 w791 w811 w814 w822 w840 w873 w961 w980 w991 w1004 w1015 w1040 w1045 w1048 w1053 w1077]
      tunnel: [w25 w178 w187 w200 errorcluster {"status"=FALSE, "code"=0, "source"=""} ("error out") w211 w216 w233 w245 w253 w274 w296 w300 w306 w338 w344 w361 w373 w400 w415 w418 w432 w437 w448 w453 w468 w473 w477 w489 w505 w522 w583 w640 w765 w773 w787 w808 w818 w823 w831 w872 w965 w981 w988 w1005 w1026 w1035 w1043 w1049 w1054 w1065] -> w18
      tunnel: w12 -> [w24 w178 w186 w200 w205 w211 w216 w233 w245 w259 w275 w294 w300 w313 w338 w344 w362 w374 w400 w415 w425 w432 w437 w448 w453 w468 w473 w477 w489 w505 w519 w580 w641 w765 w774 w793 w807 w817 w823 w826 w872 w957 w981 w987 w1005 w1026 w1036 w1044 w1049 w1055 w1067]
      tunnel: [w27 w179 w184 w202 w208 w213 w217 w235 w246 w261 w287 w297 w301 w314 w339 w351 w364 w375 w401 w416 w429 w433 w438 w449 w456 w469 w474 w478 w490 w506 w530 w589 w648 w771 w784 w805 w812 w820 w824 w841 w880 w967 w982 w992 w1006 w1027 w1041 w1046 w1050 w1060 w1078] -> w17
      tunnel: [_ _ _ _ _ TRUE _ _ _ _ _ _ _ _ _ _ _ _ _ _ _ _ _ _ _ _ _ _ _ _ _ _ _ _ _ _ _ _ _ _ _ _ _ _ _ _ _ _ _ _ _] -> w16
      tunnel: [w23 w177 w183 w201 w206 w212 w215 w234 w241 w257 w264 w293 w299 w305 w318 w349 w363 w372 w399 w414 w428 w431 w436 w447 w455 w467 w472 w476 w488 w504 w515 w574 w646 w767 w782 w792 w811 w815 w822 w839 w879 w966 w980 w990 w1004 w1014 w1040 w1045 w1048 w1052 w1077] -> w15
      tunnel: w13 -> [w22 _ _ _ _ _ _ _ _ _ _ _ _ _ _ _ _ _ _ _ _ _ _ _ _ _ _ _ _ _ _ _ _ _ _ _ _ _ _ _ _ _ _ _ _ _ _ _ _ _ _]
      tunnel: w11 -> [_ _ _ _ _ _ _ w220 _ _ _ _ _ _ _ _ _ _ _ _ _ _ _ _ _ _ _ _ _ _ _ _ _ _ _ _ _ _ _ _ _ _ _ _ _ _ _ _ _ _ _]
      tunnel: w10 -> [_ _ _ _ _ _ _ w219 _ _ _ _ _ _ _ _ _ _ _ _ _ _ _ _ _ _ _ _ _ _ _ _ _ _ _ _ _ _ _ _ _ _ _ _ _ _ _ _ _ _ _]
      frame "", "Event Structure", "Idle" {
        # "executes when the state queue is empty"
        n5 = event shown="[8] \"Lockin.Label\": Value Change" {
          selector: _ -> [_ _ _ _ _ _ _ _ _ _ _ _ _ _]
          dyn-events: _ -> [_ _ _ _ _ _ _ _ _ _ _ _ _ _]
          timeout: w22 -> [_ _ _ _ _ _ _ _ _ _ _ _ _ _]
          tunnel: w28 -> [w32 w35 w42 w48 w54 w60 w67 w73 w87 w125 w130 w149 w162 w176]
          tunnel: [w31 w37 w41 w47 w53 w59 w66 w72 w86 w125 w129 w148 w161 w175] -> w27
          tunnel: w26 -> [w29 w36 w39 w45 w51 w57 w65 w71 w85 w126 w131 w147 w159 w173]
          tunnel: [w30 w34 w40 w46 w52 w58 w62 w69 w76 w127 w132 w150 w160 w174] -> w25
          tunnel: w24 -> [w30 w34 w40 w46 w52 w58 w63 w69 w83 w127 w132 w150 w160 w174]
          tunnel: [w29 w36 w39 w45 w51 w57 w65 w71 w85 w126 w131 w147 w159 w173] -> w23
          event Timeout {
            n6 = event-data() -> ()  [unwired: 1 in, 1 out]
            n7 = call <vilib>:"Add State(s) to Queue__jki_lib_state_machine.vi"("State(s) in (\"\")"=w32) -> ("States Out"=w31:string)  [unwired: 14 in]
          }
          event "Labels Strings": Value Change {
            n8 = event-data() -> ()  [unwired: 1 in, 6 out]
            n9 = property on="Ring" class="Ring (strict)"("Strings []"="Labels Strings") -> ()  [unwired: 2 in, 2 out]
            n10 = property on="Ring" class="Ring (strict)"("Strings []"="Labels Strings") -> ()  [unwired: 2 in, 2 out]
            n11 = call <vilib>:"Add State(s) to Queue__jki_lib_state_machine.vi"("State(s) in (\"\")"=w35) -> ("States Out"=w37:string)  [unwired: 14 in]
          }
          event "OK": Value Change {
            # "Exit Button Value Change (pressed) Event\n(this executes Macro: Exit to terminate the VI)"
            n12 = event-data() -> ()  [unwired: 1 in, 1 out]
            n13 = call <vilib>:"Add State(s) to Queue__jki_lib_state_machine.vi"("State(s) in Front (\"\")"="Macro: Exit", "State(s) in (\"\")"=w42) -> ("States Out"=w41:string)  [unwired: 13 in]
          }
          event "Open VI": Value Change {
            # "Exit Button Value Change (pressed) Event\n(this executes Macro: Exit to terminate the VI)"
            n14 = event-data() -> ()  [unwired: 1 in, 6 out]
            n15 = local write "Open VI"(FALSE ("Open VI")) -> ()
            n16 = call <vilib>:"Add State(s) to Queue__jki_lib_state_machine.vi"("State(s) in Front (\"\")"="Experiment VI: Open VI", "State(s) in (\"\")"=w48) -> ("States Out"=w47:string)  [unwired: 13 in]
          }
          event "Open Lockin": Value Change {
            # "Exit Button Value Change (pressed) Event\n(this executes Macro: Exit to terminate the VI)"
            n17 = event-data() -> ()  [unwired: 1 in, 6 out]
            n18 = local write "Open Lockin"(FALSE ("Open VI")) -> ()
            n19 = call <vilib>:"Add State(s) to Queue__jki_lib_state_machine.vi"("State(s) in Front (\"\")"="Experiment VI: Open Lockin", "State(s) in (\"\")"=w54) -> ("States Out"=w53:string)  [unwired: 13 in]
          }
          event "Instrument Configuration": Value Change {
            # "Exit Button Value Change (pressed) Event\n(this executes Macro: Exit to terminate the VI)"
            n20 = event-data() -> ()  [unwired: 1 in, 6 out]
            n21 = local write "Instrument Configuration"(FALSE ("Open VI")) -> ()
            n22 = call <vilib>:"Add State(s) to Queue__jki_lib_state_machine.vi"("State(s) in Front (\"\")"="Instruments: Load Classes\nUI: View Instruments\nMetadata: Write FGV", "State(s) in (\"\")"=w60) -> ("States Out"=w59:string)  [unwired: 13 in]
          }
          event "Create Output": Value Change {
            # "\"Create Output\" Value Change (pressed) Event\n(this executes Macro: Output)"
            n23 = event-data() -> ()  [unwired: 1 in, 6 out]
            n24 = invoke on="Create Output" class="Bool" method="Reinit To Default"(error in=w63) -> (error out=w62:errorcluster)  [unwired: 2 in, 2 out]
            n25 = property on="Values have changed" class="Bool (strict)"("Val(Sgnl)"=FALSE ("Value (Signaling)")) -> ()  [unwired: 2 in, 2 out]
            n26 = call <vilib>:"Add State(s) to Queue__jki_lib_state_machine.vi"("State(s) in Front (\"\")"="Macro: Output", "State(s) in (\"\")"=w67) -> ("States Out"=w66:string)  [unwired: 13 in]
          }
          event "Values have changed": Value Change {
            # "\"Values have changed\" Value Change (pressed) Event\n(this executes Macro: Output)"
            n27 = event-data() -> ("NewVal"=w68:bool)  [unwired: 1 in, 5 out]
            n28 = property on="Values have changed" class="Bool (strict)"("Blinking"=w68) -> ()  [unwired: 2 in, 2 out]
            n29 = property on="String" class="Str"("Blinking"=w68) -> ()  [unwired: 2 in, 2 out]
            n30 = call <vilib>:"Add State(s) to Queue__jki_lib_state_machine.vi"("State(s) in Front (\"\")"="", "State(s) in (\"\")"=w73) -> ("States Out"=w72:string)  [unwired: 13 in]
          }
          event "Lockin.Label": Value Change {
            # "F: not found\nground\nT: found:\n0 - Vsg - gate\n1 - Vbg - gate\n2 - I ----- current\n????:\n4 - V ---- voltage\n3 - dV(?) voltage diff"
            # "Label Value Change Event\n(chooses proper configuration for amplifiers)"
            n31 = event-data() -> ("NewVal"=w84:u16[])  [unwired: 1 in, 5 out]
            n32 = for {
              tunnel: w84 -> [w95] mode=indexing
              tunnel: [w97] -> w80 mode=indexing
              tunnel: w83 -> [w94]
              tunnel: [w93] -> w76
              tunnel: [w92] -> w77 mode=indexing
              tunnel: [w88] -> w78 mode=indexing
              n33 = property on="Label" class="Ring (strict)"(error in=w94) -> (error out=w93:errorcluster, "Strings []"=w96:string[])  [unwired: 1 in, 1 out]
              n34 = Index Array(array=w96, index=w95) -> (element=w91:string)
              n35 = call <userlib>:"MGI String Pattern Match Exists.vi"("Patterns to Try"=string[] ["Vsg", "Vbg", "Vtg", "I", "dV", "V"], "String"=w91) -> ("Index of First Pattern Matched"=w98:i32, "Match Found"=w89:bool)
              n36 = case shown="True" w89 {
                tunnel: w98 -> [_ w105]
                tunnel: [KH_Mode-enum."Ground" ("Enum") w104] -> w97
                tunnel: [Shunt-Enum."Open" ("Shunt Resistor") w103] -> w92
                tunnel: [Input_Configuration-Enum."Ground" ("Input Configuation") w102] -> w88
                frame False {
                }
                frame True {
                  n37 = case shown="2" w105 {
                    tunnel: [KH_Mode-enum."Gate" ("Enum") KH_Mode-enum."Gate" ("Enum") KH_Mode-enum."Gate" ("Enum") KH_Mode-enum."Current" ("Enum") KH_Mode-enum."Voltage (Diff)" ("Enum") KH_Mode-enum."Voltage (SE)" ("Enum")] -> w104
                    tunnel: [Shunt-Enum."50k Ohms" ("Shunt Resistor") Shunt-Enum."50k Ohms" ("Shunt Resistor") Shunt-Enum."50k Ohms" ("Shunt Resistor") "Defualt Shunt Resistor" Shunt-Enum."Open" ("Shunt Resistor") Shunt-Enum."Open" ("Shunt Resistor")] -> w103
                    tunnel: [Input_Configuration-Enum."Differential" ("Input Configuation") Input_Configuration-Enum."Differential" ("Input Configuation") Input_Configuration-Enum."Differential" ("Input Configuation") Input_Configuration-Enum."Differential" ("Input Configuation") Input_Configuration-Enum."Differential" ("Input Configuation") Input_Configuration-Enum."SE+ (-gnd)" ("Input Configuation")] -> w102
                    frame 0, Default {
                      # "Vsg - gate"
                    }
                    frame 1 {
                      # "Vbg - gate"
                    }
                    frame 2 {
                      # "Vtg - gate"
                    }
                    frame 3 {
                      # "I - current"
                    }
                    frame 4 {
                      # "dV - V (Diff)"
                    }
                    frame 5 {
                      # "V - V (SE)"
                    }
                  }
                }
              }
            }
            n38 = property on="Values have changed" class="Bool (strict)"("Val(Sgnl)"=TRUE ("Values have changed")) -> ()  [unwired: 2 in, 2 out]
            n39 = local read "Lockin"() -> (w81:T7)
            n40 = Bundle By Name(cluster=w81, "Electrode Config"=w80) -> (w75:T7)
            n41 = local read "KH"() -> (w79:T5)
            n42 = Bundle By Name(cluster=w79, "KH Shunt Resistor"=w77, "KH Configuration"=w78) -> (w74:T5)
            n43 = local write "Lockin"(w75) -> ()
            n44 = local write "KH"(w74) -> ()
            n45 = call <vilib>:"Add State(s) to Queue__jki_lib_state_machine.vi"("State(s) in (\"\")"=w87) -> ("States Out"=w86:string)  [unwired: 14 in]
          }
          event "KH.KH Shunt Resistor", "KH.KH Gain", "non KH.Electrodes 2", "non KH.Labels 2", "Sample (SAXXXX)", "Username", "Description", "Lockin.Electrode": Value Change {
            n46 = event-data() -> ()  [unwired: 1 in, 6 out]
            n47 = property on="Values have changed" class="Bool (strict)"("Val(Sgnl)"=TRUE ("Values have changed")) -> ()  [unwired: 2 in, 2 out]
          }
          event "Lockin.AI", "non KH.Scroll Bar": Mouse Move; "Lockin.AI", "non KH.Scroll Bar": Mouse Wheel {
            n48 = event-data() -> ()  [unwired: 1 in, 5 out]
            n49 = call <vilib>:"Add State(s) to Queue__jki_lib_state_machine.vi"("State(s) in Front (\"\")"="UI: Link Scroll Bars" ("State(s) in Front (\"\")"), "State(s) in (\"\")"=w130) -> ("States Out"=w129:string)  [unwired: 13 in]
          }
          event "AI Channels": Value Change {
            n50 = event-data() -> ("NewVal"=w143:u32)  [unwired: 1 in, 5 out]
            n51 = for {
              N: w143 -> [_]
              tunnel: [w152] -> w138 mode=indexing
              tunnel: [w151] -> w134 mode=indexing
              i -> [w151]
              n52 = Increment(x=w151) -> (x+1=w152:i32)
            }
            n53 = local read "KH Addresses"() -> (w137:refnum<visa-resource-name>[])
            n54 = local read "Lockin"() -> (w146:T7)
            n55 = Empty Array?(array=w137) -> (empty?=w136:bool)
            n56 = Initialize Array(1.0 ("element"), w143) -> (w141:dbl[])
            n57 = Bundle By Name(cluster=w146, "AI"=w138) -> (w145:T7)
            n58 = Select(t=i32[] [], s=w136, f=w134) -> (s? t:f=w133:i32[])
            n59 = local read "KH"() -> (w140:T5)
            n60 = local write "Gain"(w141) -> ()
            n61 = Bundle By Name(cluster=w140, "KH #"=w133) -> (w144:T5)
            n62 = local write "Lockin"(w145) -> ()
            n63 = local write "KH"(w144) -> ()
            n64 = call <vilib>:"Add State(s) to Queue__jki_lib_state_machine.vi"("State(s) in Front (\"\")"="Metadata: Update AI\nMetadata: Update KH\nKH: set KH 0\nKH: set KH 1" ("State(s) in Front (\"\")"), "State(s) in (\"\")"=w149) -> ("States Out"=w148:string)  [unwired: 13 in]
          }
          event "KH Addresses": Value Change {
            # "?"
            n65 = event-data() -> ("NewVal"=w154:refnum<visa-resource-name>[])  [unwired: 1 in, 5 out]
            n66 = Empty Array?(array=w154) -> (empty?=w153:bool)
            n67 = local read "AI Channels"() -> (w155:u32)
            n68 = disable-structure shown="Disabled" {
              frame Disabled {
                n69 = local read "KH"() -> (w163:T5)
                n70 = Unbundle By Name(w163) -> ("KH #"=w165:u16[])
                n71 = Array Subset(array=w165) -> (w164:u16[])  [unwired: 2 in]
                n72 = Bundle By Name(cluster=w163, "KH #"=w164) -> (w166:T5)
                n73 = local write "KH"(w166) -> ()
              }
              frame Enabled {
              }
            }
            n74 = case shown="False" w153 {
              tunnel: [w167 i32[] []] -> w156
              tunnel: w155 -> [w168 _]
              frame False {
                n75 = for {
                  N: w168 -> [_]
                  tunnel: [w169] -> w167 mode=indexing
                  i -> [w169]
                }
              }
              frame True {
              }
            }
            n76 = control-ref of="KH #"() -> (w157:refnum<vi>)
            n77 = property class="Arr (strict)"(reference=w157, "Value"=w156) -> ()  [unwired: 1 in, 2 out]
            n78 = call <vilib>:"Add State(s) to Queue__jki_lib_state_machine.vi"("State(s) in Front (\"\")"="KH: set KH 0\nKH: set KH 1", "State(s) in (\"\")"=w162) -> ("States Out"=w161:string)  [unwired: 13 in]
          }
          event Panel Close? {
            # "Discard the event because we'll close the front panel ourselves in Macro: Exit"
            # "Close Panel button (pressed) Event\n(this executes Macro: Exit to terminate the VI)"
            n79 = event-data() -> ()  [unwired: 1 in, 1 out]
            n80 = event-data("Discard?"=TRUE) -> ()  [unwired: 1 in, 1 out]
            n81 = call <vilib>:"Add State(s) to Queue__jki_lib_state_machine.vi"("State(s) in Front (\"\")"="Macro: Exit", "State(s) in (\"\")"=w176) -> ("States Out"=w175:string)  [unwired: 13 in]
          }
        }
      }
      frame "---------- Core ----------" {
        # "Do not put any code in this frame.\n(it is a separator no-op)"
        n82 = call <vilib>:"Add State(s) to Queue__jki_lib_state_machine.vi"("State(s) in (\"\")"=w180) -> ("States Out"=w179:string)  [unwired: 14 in]
      }
      frame Default {
        w190 = 42 items=["No error", "Argument error", "Memory is full", "Out of zone", "End of file", "File already open", "Generic file I/O error", "File not found", "File permission error", "Disk is full", "Duplicate path", "Too many files open", "System feature not enabled", "Resource file not found", "Cannot add resource", "Resource not found", "Image not found", "Image memory error", "Pen does not exist", "Config type invalid", "Config token not found", "Config parse error", "Config memory error", "Bad external code format", "Bad external code offset", "External code not present", "Null window", "Destroy window error", "Null menu", "Print aborted", "Bad print record", "Print driver error", "Windows error during printing", "Memory error during printing", "Print dialog error", "Generic print error", "Invalid device refnum", "Device not found", "Device parameter error", "Device unit error", "Cannot open device", "Device call aborted", "Generic error", "Cancelled by user", "Object ID too low", "Object ID too high", "Object not in heap", "Unknown heap", "Unknown object (invalid DefProc)", "Unknown object (DefProc not in table)", "Message out of range", "Invalid (null) method", "Unknown message", "Manager call not supported", "Bad address", "Network operation in progress", "Network operation timed out", "Connection is busy", "Network attribute not supported", "Network error", "Address in use", "System out of memory", "Connection aborted", "Connection refused", "Not connected", "Already connected", "Connection closed", "Initialization error (interapplication manager)", "Bad occurrence", "Wait on unbound occurrence handler", "Occurrence queue overflow", "Datalog type conflict", "Unused", "Unrecognized type (interapplication manager)", "Memory corrupt", "Failed to make temporary DLL", "Old CIN version", "Drag socket not found", "Failed to load drop-object", "Failed to register OLE object", "Failed to release OLE object", "Format specifier type mismatch", "Unknown format specifier", "Too few format specifiers", "Too many format specifiers", "Scan failed", "Newer CIN version", "Error converting to variant", "Runtime menu error", "Password tampered", "Variant attribute not found", "Incompatible variant data type", "Event data is not available", "Event Store is not present", "Occurrence is not found", "Event Queue is not created", "Event info is not available", "Refnum passed is NULL", "Error retrieving Class GUID", "Error retrieving CoClass GUID", "Error retrieving TypeLib GUID.", "Bad built application magic bytes.", "Specific driver is different from the specific driver associated with the Logical Name.", "There is no session opened to the class driver.", "Max Error", "MAX - Error with config objects", "MAX - Error loading configuration", "MAX - Group not supported"]
        # "Current State"
        # "Do not delete, rename, or modify this frame.\n(this is used to capture unhandled states and typos)"
        # "Handle mistyped state name (developer tool)"
        n83 = Format Into String(format string="Software Exception: Unhandled State \"%s\"." ("message"), error in=w186, w181) -> (resulting string=w189:string, error out=w188:errorcluster)  [unwired: 1 in]
        n84 = call <vilib>:"Error Cluster From Error Code.vi"("show call chain? (False)"=TRUE, "error in (no error)"=w188, "error message (\"\")"=w189, "error code (0)"=w190) -> ("error out"=w187:errorcluster)  [unwired: 5 in]
        n85 = call <vilib>:"Add State(s) to Queue__jki_lib_state_machine.vi"("State(s) in (\"\")"=w185) -> ("States Out"=w184:string)  [unwired: 14 in]
      }
      frame "Initialize Core Data" {
        # "Do not delete, rename, or modify this frame.\n(this is used to determine panel behavior on exit)"
        # "originally closed?"
        # "exe?"
        # "If panel starts closed or is an EXE, then close it when we exit"
        n86 = property class="VI"() -> ("Front Panel.Open"=w199:bool)  [unwired: 2 in, 2 out]
        n87 = property class="App"() -> ("App.Kind"=w198:T11)  [unwired: 2 in, 2 out]
        n88 = control-ref of="Current VI Reference"() -> (w192:refnum<vi>)
        n89 = Not(x=w199) -> (.not. x?=w196:bool)
        n90 = Equal?(x=w198, y=T11."Run Time System" ("Application:Kind")) -> (x = y?=w195:bool)
        n91 = Or(x=w196, y=w195) -> (x .or. y?=w193:bool)
        n92 = Bundle By Name(cluster=w194, "Core.Current VI Reference"=w192, "Core.Close Panel on Exit?"=w193) -> (w201:T24)
        n93 = call <vilib>:"Add State(s) to Queue__jki_lib_state_machine.vi"("State(s) in (\"\")"=w203) -> ("States Out"=w202:string)  [unwired: 14 in]
      }
      frame "Error Handler" {
        # "Unhandled Error -- Display it"
        # "Handle any errors here.\nYou can also output any states to clean-up after errors occur"
        # "Clear error"
        n94 = call <vilib>:"General Error Handler.vi"("error in (no error)"=w205) -> ()  [unwired: 10 in, 5 out]
        n95 = call <vilib>:"Add State(s) to Queue__jki_lib_state_machine.vi"("State(s) in Front (\"\")"="/* Post Error States", "State(s) in (\"\")"=w209) -> ("States Out"=w208:string)  [unwired: 13 in]
      }
      frame "Exit" {
        # "Do not put any code in this frame.\n(No errors that occur here will be handled.)"
        n96 = call <vilib>:"Add State(s) to Queue__jki_lib_state_machine.vi"("State(s) in (\"\")"=w214) -> ("States Out"=w213:string)  [unwired: 14 in]
      }
      frame "---------- Data ----------" {
        # "Do not put any code in this frame.\n(It is a separator no-op. You can make a copy of this frame to create a new Data frame)"
        n97 = call <vilib>:"Add State(s) to Queue__jki_lib_state_machine.vi"("State(s) in (\"\")"=w218) -> ("States Out"=w217:string)  [unwired: 14 in]
      }
      frame "Data: Initialize" {
        w221 = FALSE  # top level?
        w222 = path[] []  # VI paths
        w223 = refnum<class "Logger.PGSQL.lvclass"> refnum  # Logger
        w224 = T23 {"Sample"="", "Device"="", "Username"="", "Description"="", "Default Path"=path "", "AWS Path"=path "", "Instrument"=enum."----- AFM/EBL -----", "Lockin?"=FALSE, "Lockin Address"="", "Krohn Hite?"=FALSE, "KH Addresses"=[], "KH All Buttons"=enum."No Selection", "Strain Cell?"=FALSE, "Strain Cell Address"="", "C Bridge?"=FALSE, "Capacitance Bridge Address"="", "Lockin"={"AI"=[], "Electrode"=[], "Label"=[], "Electrode Config"=[]}, "KH"={"KH #"=[], "KH Configuration"=[], "KH Gain"=[], "KH Shunt Resistor"=[], "Filter"=FALSE, "DC Coupled"=FALSE}, "non KH"={"Scroll Bar"=[], "Electrodes 2"=[], "Labels 2"=[], "unused"=[]}}  # UI
        w228 = refnum<class "Configuration.lvclass"> refnum  # Config
        w230 = cluster{"Channel Setting":T22}[] []  # Channel Settings
        w226 = T25 {"Current VI Reference"=refnum, "Close Panel on Exit?"=FALSE}  # Core
        # "Initialize the shift-register data, here.\n(data names are defined by what you wire into the bundle function)"
        n98 = Unbundle By Name("C.E.") -> ("Experiment"=w231:T19, "Wiring Configuration"=w232:T21)
        n99 = Bundle("Core"=w226, "C.E."="C.E.", "Experiment"=w231, "Wiring Configuration"=w232, "Channel Settings"=w230, "KH All Buttons"="KH All Buttons", "Lockin"=w220, "KH"=w219, "non KH"="non KH", "UI"=w224, "Logger"=w223, "Config"=w228, "VI paths"=w222, "top level?"=w221) -> (w234:T24)  [unwired: 1 in]
        n100 = call <vilib>:"Add State(s) to Queue__jki_lib_state_machine.vi"("State(s) in (\"\")"=w236) -> ("States Out"=w235:string)  [unwired: 14 in]
      }
      frame "Data: Initialize Top Level" {
        # "Do not put any code in this frame.\n(It is a separator no-op. You can make a copy of this frame to create a new Data frame)"
        n101 = property class="VI"() -> ("Exec.State"=w244:T12)  [unwired: 2 in, 2 out]
        n102 = Equal?(x=w244, y=T12."Run top level" ("Execution:State")) -> (x = y?=w240:bool)
        n103 = Select(t="", s=w240, f="Macro: Output\nMacro: Exit") -> (s? t:f=w239:string)
        n104 = Bundle By Name(cluster=w242, "top level?"=w240) -> (w241:T24)
        n105 = call <vilib>:"Add State(s) to Queue__jki_lib_state_machine.vi"("State(s) in (\"\")"=w247, "State(s) at Back (\"\")"=w239) -> ("States Out"=w246:string)  [unwired: 13 in]
      }
      frame "Data: Load Configuration" {
        n106 = Unbundle By Name(w258) -> ("Config"=w260:refnum<class "Configuration.lvclass">, "UI"=w252:T23)
        n107 = call <userlib>:"Default Path.vi"("error in (no error)"=w259, "Folder Name [Application Name]"="Control Experiment" ("name or relative path"), "Configuration in"=w260) -> ("error out"=w255:errorcluster, "Configuration out"=w256:refnum<class "Configuration.lvclass">)  [unwired: 7 in]
        n108 = call <userlib>:"Read Configuration.vi"("INI Fomatted Cluster Type"=w252, "error in (no error)"=w255, "Configuration in"=w256) -> ("error out"=w254:errorcluster, "Configuration"=w250:variant, "Configuration out"=w251:refnum<class "Configuration.lvclass">)  [unwired: 6 in]
        n109 = Variant To Data(error in=w254, type=w252, Variant=w250) -> (data=w248:T23, error out=w253:errorcluster)
        n110 = Bundle By Name(cluster=w258, "Config"=w251, "UI"=w248) -> (w257:T24)
        n111 = call <vilib>:"Add State(s) to Queue__jki_lib_state_machine.vi"("State(s) in (\"\")"=w262) -> ("States Out"=w261:string)  [unwired: 14 in]
      }
      frame "Data: Save Controls" {
        n112 = local read "Sample (SAXXXX)"() -> (w286:string)
        n113 = local read "Lockin"() -> (w278:T7)
        n114 = local read "Username"() -> (w284:string)
        n115 = local read "Default Path"() -> (w282:path)
        n116 = local read "KH Addresses"() -> (w280:refnum<visa-resource-name>[])
        n117 = local read "KH"() -> (w271:T5)
        n118 = local read "Description"() -> (w283:string)
        n119 = Unbundle By Name(w271) -> ("KH #"=w270:u16[], "KH Configuration"=w267:T2[], "KH Gain"=w268:T3[], "KH Shunt Resistor"=w269:T4[])
        n120 = local read "Instrument"() -> (w281:T9)
        n121 = local read "Device (YYYYMMDD)"() -> (w285:string)
        n122 = local read "KH All Buttons"() -> (w279:T8)
        n123 = local read "non KH"() -> (w272:T10)
        n124 = Bundle By Name(cluster=w273, "UI.Sample"=w286, "UI.Device"=w285, "UI.Username"=w284, "UI.Description"=w283, "UI.Default Path"=w282, "UI.AWS Path"=path "", "UI.Instrument"=w281, "UI.KH Addresses"=w280, "UI.KH All Buttons"=w279, "UI.Lockin"=w278, "UI.non KH"=w272, "UI.KH.KH #"=w270, "UI.KH.KH Configuration"=w267, "UI.KH.KH Gain"=w268, "UI.KH.KH Shunt Resistor"=w269, "UI.KH.Filter"="Bandwidth Filter", "UI.KH.DC Coupled"="DC Coupled") -> (w264:T24)
        n125 = Unbundle By Name(w264) -> ("Config"=w277:refnum<class "Configuration.lvclass">, "UI"=w276:T23)
        n126 = call <userlib>:"Write Configuration.vi"("error in (no error)"=w275, "Variant"=w276, "Configuration in"=w277) -> ("error out"=w274:errorcluster)  [unwired: 7 in, 1 out]
        n127 = call <vilib>:"Add State(s) to Queue__jki_lib_state_machine.vi"("State(s) in (\"\")"=w288) -> ("States Out"=w287:string)  [unwired: 14 in]
      }
      frame "Data: Cleanup" {
        # "Cleanup any data and references, here.\n(this is called automatically, by the Macro: Exit)"
        n128 = Unbundle By Name(w293) -> ("Core.Current VI Reference"=w292:refnum<vi>, "Logger"=w295:refnum<class "Logger.PGSQL.lvclass">)
        n129 = call <vilib>:"Stop.vi"("error in (no error)"=w294, "SMO"=w295) -> ("error out"=w290:errorcluster, "SMO out"=w291:refnum<class "Logger.PGSQL.lvclass">)  [unwired: 8 in]
        n130 = call <vilib>:"Destroy.vi"("error in (no error)"=w290, "SMO"=w291) -> ("error out"=w289:errorcluster)  [unwired: 9 in]
        n131 = Close Reference(reference=w292, error in (no error)=w289) -> (error out=w296:errorcluster)
        n132 = call <vilib>:"Add State(s) to Queue__jki_lib_state_machine.vi"("State(s) in (\"\")"=w298) -> ("States Out"=w297:string)  [unwired: 14 in]
      }
      frame "---------- UI ----------" {
        # "Do not put any code in this frame.\n(It is a separator no-op. You can make a copy of this frame to create a new UI frame)"
        n133 = call <vilib>:"Add State(s) to Queue__jki_lib_state_machine.vi"("State(s) in (\"\")"=w302) -> ("States Out"=w301:string)  [unwired: 14 in]
      }
      frame "UI: Initialize" {
        (unwired) string[] ["", "I+", "I-", "V1+", "V1-", "V2+", "V2-", "V3+", "V3-", "V4+", "V4-", "dV1", "dV2", "dV3", "Vsg", "Vbg", "Vtg"] ("Strings [] 2")
        # "Initialize the User Interface, here.\n(this is called automatically, by the Macro: Init)"
        n134 = local read "Labels Strings"() -> (w309:string[])
        n135 = call <userlib>:"Fit VI window to Largest Dec__ogtk.vi"("error in (no error)"=w313) -> ("error out"=w311:errorcluster)  [unwired: 5 in, 1 out]
        n136 = Unbundle By Name(w305) -> ("top level?"=w303:bool)
        n137 = property on="OK" class="Bool (strict)"("Value"=FALSE ("Blinking")) -> ()  [unwired: 2 in, 2 out]
        n138 = property on="Tab Control" class="TabCtl (strict)"("Value"=T1."Input" ("Tab Control")) -> ()  [unwired: 2 in, 2 out]
        n139 = property on="Ring" class="Ring (strict)"(error in=w311, "Strings []"=w309) -> (error out=w310:errorcluster)  [unwired: 1 in, 1 out]
        n140 = local write "KH All Buttons"(T8."No Selection" ("KH All Buttons")) -> ()
        n141 = property on="Values have changed" class="Bool (strict)"("Val(Sgnl)"=TRUE ("Blinking")) -> ()  [unwired: 2 in, 2 out]
        n142 = property on="Ring" class="Ring (strict)"(error in=w310, "Strings []"=w309) -> (error out=w306:errorcluster)  [unwired: 1 in, 1 out]
        n143 = case shown="True" w303 {
          frame False {
          }
          frame True {
            # "unused"
            n144 = local read "KH Addresses"() -> (w316:refnum<visa-resource-name>[])
            n145 = property on="AI Channels" class="DigNum (strict)"("Val(Sgnl)"="AI Channels") -> ()  [unwired: 2 in, 2 out]
            n146 = property on="KH Addresses" class="Arr (strict)"("Val(Sgnl)"=w316) -> ()  [unwired: 2 in, 2 out]
          }
        }
        n147 = call <vilib>:"Add State(s) to Queue__jki_lib_state_machine.vi"("State(s) in (\"\")"=w315) -> ("States Out"=w314:string)  [unwired: 14 in]
      }
      frame "UI: Update Controls" {
        # "Do not put any code in this frame.\n(It is a separator no-op. You can make a copy of this frame to create a new Data frame)"
        n148 = Unbundle By Name(w318) -> ("top level?"=w319:bool, "UI.Sample"=w332:string, "UI.Device"=w333:string, "UI.Username"=w334:string, "UI.Description"=w335:string, "UI.Default Path"=w337:path, "UI.Instrument"=w336:T9, "UI.KH Addresses"=w331:refnum<visa-resource-name>[], "UI.KH All Buttons"=w330:T8, "UI.Lockin"=w321:T7, "UI.non KH"=w320:T10, "UI.KH.Filter"=w328:bool, "UI.KH.DC Coupled"=w329:bool, "UI.KH.KH #"=w325:T26, "UI.KH.KH Configuration"=w324:T2[], "UI.KH.KH Gain"=w323:T3[], "UI.KH.KH Shunt Resistor"=w322:T4[])  [unwired: 2 out]
        n149 = local write "Sample (SAXXXX)"(w332) -> ()
        n150 = local write "Username"(w334) -> ()
        n151 = local write "Instrument"(w336) -> ()
        n152 = local write "Default Path"(w337) -> ()
        n153 = local write "KH Addresses"(w331) -> ()
        n154 = local write "Bandwidth Filter"(w328) -> ()
        n155 = local write "DC Coupled"(w329) -> ()
        n156 = local write "Device (YYYYMMDD)"(w333) -> ()
        n157 = local write "Description"(w335) -> ()
        n158 = local write "KH All Buttons"(w330) -> ()
        n159 = local read "KH"() -> (w327:T5)
        n160 = Bundle By Name(cluster=w327, "KH #"=w325, "KH Configuration"=w324, "KH Gain"=w323, "KH Shunt Resistor"=w322) -> (w326:T5)
        n161 = case shown="True" w319 {
          tunnel: w326 -> [_ w343]
          tunnel: w321 -> [_ w342]
          tunnel: w320 -> [_ w341]
          frame False {
          }
          frame True {
            n162 = local write "non KH"(w341) -> ()
            n163 = local write "Lockin"(w342) -> ()
            n164 = local write "KH"(w343) -> ()
          }
        }
        n165 = call <vilib>:"Add State(s) to Queue__jki_lib_state_machine.vi"("State(s) in (\"\")"=w340) -> ("States Out"=w339:string)  [unwired: 14 in]
      }
      frame "UI: View Instruments" {
        n166 = Unbundle By Name(w349) -> ("C.E."=w350:refnum<class "Control Experiment.lvclass">)
        n167 = Unbundle By Name(w350) -> ("Instruments"=w348:T27)
        n168 = for {
          tunnel: w348 -> [w359] mode=indexing
          tunnel: [w353] -> w347 mode=indexing
          n169 = Unbundle By Name(w359) -> ("Type"=w356:T20, "class path"=w358:path, "Address"=w354:string)
          n170 = Strip Path(path=w358) -> (name=w355:string)  [unwired: 1 out]
          n171 = Format Into String(format string="%s:\n- %s\n- %s", w356, w355, w354) -> (resulting string=w353:string)  [unwired: 2 in, 1 out]
        }
        n172 = call <vilib>:"1D String Array to Delimited String.vi"("delimiter"="\n", "string array"=w347) -> ("delimited string"=→"Instruments":string)  [unwired: 9 in]
        n173 = call <vilib>:"Add State(s) to Queue__jki_lib_state_machine.vi"("State(s) in (\"\")"=w352) -> ("States Out"=w351:string)  [unwired: 14 in]
      }
      frame "UI: Cursor Set" {
        # "Argument"
        # "Set and Unset Cursor Busy.\n(Usage: \"UI: Cursor Set >> Busy|Idle\")"
        n174 = case shown="\"Busy\"" w360 {
          tunnel: w362 -> [w367 w369]
          tunnel: [w366 w368] -> w361
          frame "Idle", Default {
            n175 = call <vilib>:"Unset Busy.vi"("error in (no error)"=w367) -> ("error out"=w366:errorcluster)  [unwired: 10 in]
          }
          frame "Busy" {
            n176 = call <vilib>:"Set Busy.vi"("error in (no error)"=w369) -> ("error out"=w368:errorcluster)  [unwired: 9 in, 1 out]
          }
        }
        n177 = call <vilib>:"Add State(s) to Queue__jki_lib_state_machine.vi"("State(s) in (\"\")"=w365) -> ("States Out"=w364:string)  [unwired: 14 in]
      }
      frame "UI: Front Panel State" {
        # "Argument"
        # "Set Front Panel Open or Closed\n(Usage: \"UI: Front Panel State >> Open|Close\")"
        n178 = Unbundle By Name(w372) -> ("Core.Current VI Reference"=w371:refnum<vi>)
        n179 = case shown="\"Open\", Default" w370 {
          tunnel: w374 -> [w380 w393]
          tunnel: [w382 w394] -> w373
          tunnel: w371 -> [w381 w391]
          frame "Open", Default {
            n180 = property class="VI"(reference=w381, error in=w380) -> (reference out=w378:refnum<vi>, error out=w379:errorcluster, "Front Panel.Open"=w377:bool)
            n181 = case shown="True" w377 {
              tunnel: [w385 w388] -> w382
              tunnel: w379 -> [w384 w388]
              tunnel: w378 -> [w383 _]
              frame False {
                n182 = invoke class="VI" method="FP.Open"(reference=w383, error in=w384, "Activate"=TRUE, "State"=T13."Standard") -> (error out=w385:errorcluster)  [unwired: 1 in, 4 out]
              }
              frame True {
              }
            }
          }
          frame "Close" {
            n183 = property class="VI"(reference=w391, error in=w393) -> (reference out=w390:refnum<vi>, error out=w392:errorcluster, "Front Panel.Open"=w389:bool)
            n184 = case shown="True" w389 {
              tunnel: [w395 w398] -> w394
              tunnel: w392 -> [w395 w397]
              tunnel: w390 -> [_ w396]
              frame False {
              }
              frame True {
                n185 = invoke class="VI" method="FP.Close"(reference=w396, error in=w397) -> (error out=w398:errorcluster)  [unwired: 1 in, 2 out]
              }
            }
          }
        }
        n186 = call <vilib>:"Add State(s) to Queue__jki_lib_state_machine.vi"("State(s) in (\"\")"=w376) -> ("States Out"=w375:string)  [unwired: 14 in]
      }
      frame "UI: Buttons" {
        # "Do not put any code in this frame.\n(It is a separator no-op. You can make a copy of this frame to create a new UI frame)"
        n187 = call <vilib>:"Add State(s) to Queue__jki_lib_state_machine.vi"("State(s) in (\"\")"=w402) -> ("States Out"=w401:string)  [unwired: 14 in]
      }
      frame "UI: Link Scroll Bars" {
        # "Do not put any code in this frame.\n(It is a separator no-op. You can make a copy of this frame to create a new UI frame)"
        n188 = control-ref of="AI"() -> (w413:refnum<vi>)
        n189 = control-ref of="Electrode"() -> (w412:refnum<vi>)
        n190 = control-ref of="Label"() -> (w411:refnum<vi>)
        n191 = control-ref of="Electrode Config"() -> (w410:refnum<vi>)
        n192 = control-ref of="KH #"() -> (w409:refnum<vi>)
        n193 = control-ref of="KH Configuration"() -> (w408:refnum<vi>)
        n194 = control-ref of="KH Gain"() -> (w407:refnum<vi>)
        n195 = control-ref of="KH Shunt Resistor"() -> (w406:refnum<vi>)
        n196 = control-ref of="Gain"() -> (w404:refnum<vi>)
        n197 = property class="Arr (strict)"(reference=w413) -> ("Index Values"=w403:u32[])  [unwired: 1 in, 2 out]
        n198 = property class="Arr (strict)"(reference=w412, "Index Values"=w403) -> ()  [unwired: 1 in, 2 out]
        n199 = property class="Arr (strict)"(reference=w411, "Index Values"=w403) -> ()  [unwired: 1 in, 2 out]
        n200 = property class="Arr (strict)"(reference=w410, "Index Values"=w403) -> ()  [unwired: 1 in, 2 out]
        n201 = property class="Arr (strict)"(reference=w409, "Index Values"=w403) -> ()  [unwired: 1 in, 2 out]
        n202 = property class="Arr (strict)"(reference=w408, "Index Values"=w403) -> ()  [unwired: 1 in, 2 out]
        n203 = property class="Arr (strict)"(reference=w407, "Index Values"=w403) -> ()  [unwired: 1 in, 2 out]
        n204 = property class="Arr (strict)"(reference=w406, "Index Values"=w403) -> ()  [unwired: 1 in, 2 out]
        n205 = property class="Arr (strict)"(reference=w404, "Index Values"=w403) -> ()  [unwired: 1 in, 2 out]
        n206 = property on="Scroll Bar" class="Arr (strict)"() -> ("Index Values"=w405:u32[])  [unwired: 2 in, 2 out]
        n207 = property on="Labels 2" class="Arr (strict)"("Index Values"=w405) -> ()  [unwired: 2 in, 2 out]
        n208 = property on="unused" class="Arr (strict)"("Index Values"=w405) -> ()  [unwired: 2 in, 2 out]
        n209 = property on="Electrodes 2" class="Arr (strict)"("Index Values"=w405) -> ()  [unwired: 2 in, 2 out]
        n210 = call <vilib>:"Add State(s) to Queue__jki_lib_state_machine.vi"("State(s) in (\"\")"=w417) -> ("States Out"=w416:string)  [unwired: 14 in]
      }
      frame "UI: SR Disable" {
        # "Do not put any code in this frame.\n(It is a separator no-op. You can make a copy of this frame to create a new UI frame)"
        n211 = local read "KH Addresses"() -> (w427:refnum<visa-resource-name>[])
        n212 = control-ref of="Shunt Resistor"() -> (w423:refnum<vi>)
        n213 = Index Array(array=w427) -> (element=w426:refnum<visa-resource-name>)  [unwired: 1 in]
        n214 = call <userlib>:"Shunt - Check 500 or 10M.vi"("error in (no error)"=w425, "VISA Refnum in"=w426) -> ("error out"=w424:errorcluster, "SR"=w420:enum16{"500", "10M"})  [unwired: 7 in, 1 out]
        n215 = call <vilib>:"Clear Errors.vi"("error in (no error)"=w424) -> ("error out"=w422:errorcluster)  [unwired: 5 in, 1 out]
        n216 = call <userlib>:"Shunt - 500 or 10M Control Disable.vi"("error in"=w422, "SR"=w420, "reference"=w423) -> ("error out"=w419:errorcluster)  [unwired: 8 in]
        n217 = control-ref of="Defualt Shunt Resistor"() -> (w421:refnum<vi>)
        n218 = call <userlib>:"Shunt - 500 or 10M Control Disable.vi"("error in"=w419, "SR"=w420, "reference"=w421) -> ("error out"=w418:errorcluster)  [unwired: 8 in]
        n219 = call <vilib>:"Add State(s) to Queue__jki_lib_state_machine.vi"("State(s) in (\"\")"=w430) -> ("States Out"=w429:string)  [unwired: 14 in]
      }
      frame "---------- Macro ----------" {
        # "Do not put any code in this frame.\n(It is a separator no-op. You can make a copy of this frame to create a new Macro frame)"
        n220 = call <vilib>:"Add State(s) to Queue__jki_lib_state_machine.vi"("State(s) in (\"\")"=w434) -> ("States Out"=w433:string)  [unwired: 14 in]
      }
      frame "Macro: Initialize" {
        # "Initialization Macro\n(This is called once, when the VI starts)"
        n221 = call <vilib>:"Add State(s) to Queue__jki_lib_state_machine.vi"("State(s) in Front (\"\")"="Data: Initialize\nInitialize Core Data\nData: Initialize Top Level\nData: Load Configuration\nMetadata: Read FGV\nUI: View Instruments\nUI: Update Controls\nUI: Initialize\nUI: Front Panel State >> Open\nUI: SR Disable\nExperiment VI: Populate VI Ring\nPGSQL: Start Logger", "State(s) in (\"\")"=w439) -> ("States Out"=w438:string)  [unwired: 13 in]
      }
      frame "Macro: Exit" {
        # "Exit Macro\n(This is called once, when the VI exits)"
        n222 = Unbundle By Name(w447) -> ("Core.Close Panel on Exit?"=w446:bool)
        n223 = property on="OK" class="Bool (strict)"("Value"=FALSE ("Blinking")) -> ()  [unwired: 2 in, 2 out]
        n224 = Select(t="UI: Front Panel State >> Close", s=w446, f="") -> (s? t:f=w443:string)
        n225 = call <vilib>:"Add State(s) to Queue__jki_lib_state_machine.vi"("State(s) in (\"\")"=w443, "State(s) at Back (\"\")"="Data: Save Controls\nData: Cleanup\nExit") -> ("States Out"=w441:string)  [unwired: 13 in]
        n226 = call <vilib>:"Add State(s) to Queue__jki_lib_state_machine.vi"("State(s) in Front (\"\")"=w441, "State(s) in (\"\")"=w450) -> ("States Out"=w449:string)  [unwired: 13 in]
      }
      frame "Macro: Output" {
        n227 = case shown="False" "I'm Finished Taking Data!" {
          tunnel: [w465 _] -> w454
          frame False {
            n228 = local read "KH Addresses"() -> (w461:refnum<visa-resource-name>[])
            n229 = Empty Array?(array=w461) -> (empty?=w460:bool)
            n230 = Select(t="", s=w460, f="UI: SR Disable\nKH: set KH 0\nKH: set KH 1\nKH: set KH 2" ("State(s) in Front (\"\")")) -> (s? t:f=w462:string)
            n231 = call <vilib>:"Add State(s) to Queue__jki_lib_state_machine.vi"("State(s) in Front (\"\")"="Macro: Initialize Metadata" ("State(s) in Front (\"\")"), "State(s) in (\"\")"=w462, "State(s) at Back (\"\")"="Macro: Write Metadata" ("State(s) in Front (\"\")")) -> ("States Out"=w465:string)  [unwired: 12 in]
          }
          frame True {
          }
        }
        n232 = call <vilib>:"Add State(s) to Queue__jki_lib_state_machine.vi"("State(s) in Front (\"\")"=w454, "State(s) in (\"\")"=w457, "State(s) at Back (\"\")"="PGSQL: Write" ("State(s) in Front (\"\")")) -> ("States Out"=w456:string)  [unwired: 12 in]
      }
      frame "Macro: Initialize Metadata" {
        # "Do not put any code in this frame.\n(It is a separator no-op. You can make a copy of this frame to create a new Macro frame)"
        n233 = call <vilib>:"Add State(s) to Queue__jki_lib_state_machine.vi"("State(s) in Front (\"\")"="Metadata: Update Experiment Description\nMetadata: Update Wiring Configuration\nMetadata: Update KH\nMetadata: Build Path\nMetadata: Update Control Experiment Wire\n// Instruments: Load Classes\n// nstruments: Initialize KH" ("State(s) in Front (\"\")"), "State(s) in (\"\")"=w470) -> ("States Out"=w469:string)  [unwired: 13 in]
      }
      frame "Macro: Write Metadata" {
        # "Do not put any code in this frame.\n(It is a separator no-op. You can make a copy of this frame to create a new Macro frame)"
        n234 = call <vilib>:"Add State(s) to Queue__jki_lib_state_machine.vi"("State(s) in Front (\"\")"="Metadata: Update Comments\nMetadata: Write JSON\nMetadata: Write FGV" ("State(s) in Front (\"\")"), "State(s) in (\"\")"=w475) -> ("States Out"=w474:string)  [unwired: 13 in]
      }
      frame "---------- Metadata ----------" {
        n235 = call <vilib>:"Add State(s) to Queue__jki_lib_state_machine.vi"("State(s) in (\"\")"=w479) -> ("States Out"=w478:string)  [unwired: 14 in]
      }
      frame "Metadata: Update Experiment Description" {
        n236 = Concatenate Strings("Sample (SAXXXX)", "." ("string"), "Device (YYYYMMDD)") -> (w483:string)
        n237 = Bundle By Name(cluster=w487, "Experiment.Device"=w483, "Experiment.User"="Username", "Experiment.Device Description"="Description", "Experiment.Instrument"="Instrument") -> (w488:T24)
        n238 = call <vilib>:"Add State(s) to Queue__jki_lib_state_machine.vi"("State(s) in (\"\")"=w491) -> ("States Out"=w490:string)  [unwired: 14 in]
      }
      frame "Metadata: Update Wiring Configuration" {
        n239 = local read "Lockin"() -> (w500:T7)
        n240 = local read "non KH"() -> (w494:T10)
        n241 = local read "Lockin"() -> (w498:T7)
        n242 = Unbundle By Name(w494) -> ("Electrodes 2"=w493:string[], "Labels 2"=w492:u16[])
        n243 = Unbundle By Name(w498) -> ("Electrode Config"=w497:T6[])
        n244 = Unbundle By Name(w500) -> ("AI"=w495:u32[], "Electrode"=w496:string[], "Label"=w499:u16[])
        n245 = for {
          tunnel: w492 -> [w509] mode=indexing
          tunnel: [w508] -> w501 mode=indexing
          n246 = property on="Ring" class="Ring (strict)"() -> ("Strings []"=w510:string[])  [unwired: 2 in, 2 out]
          n247 = Index Array(array=w510, index=w509) -> (element=w508:string)
        }
        n248 = for {
          tunnel: w499 -> [w512] mode=indexing
          tunnel: [w511] -> w502 mode=indexing
          n249 = property on="Ring" class="Ring (strict)"() -> ("Strings []"=w513:string[])  [unwired: 2 in, 2 out]
          n250 = Index Array(array=w513, index=w512) -> (element=w511:string)
        }
        n251 = Bundle By Name(cluster=w503, "Wiring Configuration.Lockin Ch"=w495, "Wiring Configuration.KH.Electrodes"=w496, "Wiring Configuration.KH.Labels"=w502, "Wiring Configuration.not KH.Electrodes"=w493, "Wiring Configuration.not KH.Labels"=w501, "Lockin.Electrode Config"=w497) -> (w504:T24)
        n252 = call <vilib>:"Add State(s) to Queue__jki_lib_state_machine.vi"("State(s) in (\"\")"=w507) -> ("States Out"=w506:string)  [unwired: 14 in]
      }
      frame "Metadata: Update KH" {
        n253 = local read "KH"() -> (w528:T5)
        n254 = Unbundle By Name(w528) -> ("KH Gain"=w520:T3[], "KH Configuration"=w525:T2[], "KH Shunt Resistor"=w524:T4[], "KH #"=w517:u16[])
        n255 = Empty Array?(array=w517) -> (empty?=w518:bool)
        n256 = case shown="True" w518 {
          tunnel: [w541 w572] -> w527
          tunnel: w525 -> [w540 _]
          tunnel: w524 -> [w539 _]
          tunnel: [w538 w570] -> w523
          tunnel: w517 -> [w534 _]
          tunnel: [w537 w573] -> w522
          tunnel: [w536 w571] -> w521
          tunnel: w520 -> [w533 _]
          tunnel: w519 -> [w535 w573]
          tunnel: [w534 u16[] [] ("KH #")] -> w516
          frame False {
            n257 = Empty Array?(array=w533) -> (empty?=w532:bool)
            n258 = case shown="True" w532 {
              tunnel: [w556 w560] -> w541
              tunnel: w540 -> [w552 w562]
              tunnel: w539 -> [w551 w563]
              tunnel: [w550 w558] -> w538
              tunnel: [w549 w557] -> w537
              tunnel: [w548 w559] -> w536
              tunnel: w535 -> [w547 w557]
              tunnel: w533 -> [w543 w561]
              tunnel: w534 -> [w542 w564]
              frame False {
                n259 = call "Initialize KH Array.vi"("KH #"=w542, "Control in"=w543) -> ("Control out"=w555:variant)  [unwired: 9 in]
                n260 = call "Initialize KH Array.vi"("KH #"=w542, "Control in"=w552) -> ("Control out"=w554:variant)  [unwired: 9 in]
                n261 = call "Initialize KH Array.vi"("KH #"=w542, "Control in"=w551) -> ("Control out"=w553:variant)  [unwired: 9 in]
                n262 = Variant To Data(error in=w547, type=w543, Variant=w555) -> (data=w556:T3[], error out=w546:errorcluster)
                n263 = Variant To Data(error in=w547, type=w552, Variant=w554) -> (data=w548:T2[], error out=w545:errorcluster)
                n264 = Variant To Data(error in=w547, type=w551, Variant=w553) -> (data=w550:T4[], error out=w544:errorcluster)
                n265 = Merge Errors(w546, w545, w544) -> (w549:errorcluster)
              }
              frame True {
                n266 = Array Size(array=w564) -> (size(s)=w565:i32)
                n267 = Index Array(array=w562) -> (element=w567:T2)  [unwired: 1 in]
                n268 = Index Array(array=w563) -> (element=w566:T4)  [unwired: 1 in]
                n269 = Index Array(array=w561) -> (element=w568:T3)  [unwired: 1 in]
                n270 = Initialize Array(w568, w565) -> (w560:T3[])
                n271 = Initialize Array(w567, w565) -> (w559:T2[])
                n272 = Initialize Array(w566, w565) -> (w558:T4[])
              }
            }
          }
          frame True {
            w570 = T4[] [] items=["Open", "50 Ohms", "500 Ohms", "5k Ohms", "50k Ohms", "10M Ohm"] ("KH Shunt Resistor")
            w571 = T2[] [] items=["Ground", "SE+ (-gnd)", "SE- (+gnd)", "Differential"] ("KH Configuration")
            w572 = T3[] [] items=["1x", "10x", "100x", "1000x"] ("KH Gain")
          }
        }
        n273 = local read "KH All Buttons"() -> (w526:T8)
        n274 = Bundle By Name(cluster=w529, "KH All Buttons"=w526, "KH.KH Gain"=w527, "KH.KH Configuration"=w521, "KH.KH Shunt Resistor"=w523, "KH.KH #"=w516) -> (w515:T24)
        n275 = Unbundle By Name(w515) -> ("KH"=w514:T5)
        n276 = local write "KH"(w514) -> ()
        n277 = call <vilib>:"Add State(s) to Queue__jki_lib_state_machine.vi"("State(s) in (\"\")"=w531) -> ("States Out"=w530:string)  [unwired: 14 in]
      }
      frame "Metadata: Update AI" {
        n278 = local read "Lockin"() -> (w576:T7)
        n279 = Unbundle By Name(w576) -> ("Electrode"=w581:string[], "Label"=w586:u16[], "Electrode Config"=w585:T6[], "AI"=w578:u32[])
        n280 = Empty Array?(array=w578) -> (empty?=w579:bool)
        n281 = case shown="False" w579 {
          tunnel: [w600 string[] [] ("Electrode")] -> w587
          tunnel: w586 -> [w592 _]
          tunnel: w585 -> [w599 _]
          tunnel: [w598 w629] -> w584
          tunnel: w578 -> [w594 _]
          tunnel: [w593 w632] -> w583
          tunnel: [w597 u16[] [] ("Label")] -> w582
          tunnel: w581 -> [w595 _]
          tunnel: w580 -> [w596 w632]
          tunnel: [w594 u32[] [] ("AI")] -> w577
          frame False {
            n282 = Empty Array?(array=w592) -> (empty?=w591:bool)
            n283 = case shown="True" w591 {
              tunnel: [w615 w624] -> w600
              tunnel: w592 -> [w611 w625]
              tunnel: w599 -> [w610 w626]
              tunnel: [w609 w619] -> w598
              tunnel: [w608 w621] -> w597
              tunnel: w596 -> [w607 w616]
              tunnel: w595 -> [w603 w627]
              tunnel: w594 -> [w602 w618]
              tunnel: [w601 w616] -> w593
              frame False {
                n284 = call "Initialize KH Array.vi"("KH #"=w602, "Control in"=w603) -> ("Control out"=w614:variant)  [unwired: 9 in]
                n285 = call "Initialize KH Array.vi"("KH #"=w602, "Control in"=w611) -> ("Control out"=w613:variant)  [unwired: 9 in]
                n286 = call "Initialize KH Array.vi"("KH #"=w602, "Control in"=w610) -> ("Control out"=w612:variant)  [unwired: 9 in]
                n287 = Variant To Data(error in=w607, type=w603, Variant=w614) -> (data=w615:string[], error out=w606:errorcluster)
                n288 = Variant To Data(error in=w607, type=w611, Variant=w613) -> (data=w608:u16[], error out=w605:errorcluster)
                n289 = Variant To Data(error in=w607, type=w610, Variant=w612) -> (data=w609:T6[], error out=w604:errorcluster)
                n290 = Merge Errors(w606, w605, w604) -> (w601:errorcluster)
              }
              frame True {
                n291 = Array Size(array=w618) -> (size(s)=w617:i32)
                n292 = Index Array(array=w625) -> (element=w622:u16)  [unwired: 1 in]
                n293 = Index Array(array=w626) -> (element=w620:T6)  [unwired: 1 in]
                n294 = Index Array(array=w627) -> (element=w623:string)  [unwired: 1 in]
                n295 = Initialize Array(w623, w617) -> (w624:string[])
                n296 = Initialize Array(w622, w617) -> (w621:u16[])
                n297 = Initialize Array(w620, w617) -> (w619:T6[])
              }
            }
          }
          frame True {
            w629 = T6[] [] items=["Ground", "Current", "Voltage (SE)", "Voltage (Diff)", "Gate"] ("Electrode Config")
          }
        }
        n298 = Bundle By Name(cluster=w588, "Lockin.Electrode"=w587, "Lockin.Label"=w582, "Lockin.Electrode Config"=w584, "Lockin.AI"=w577) -> (w574:T24)
        n299 = Unbundle By Name(w574) -> ("Lockin"=w575:T7)
        n300 = local write "Lockin"(w575) -> ()
        n301 = call <vilib>:"Add State(s) to Queue__jki_lib_state_machine.vi"("State(s) in (\"\")"=w590) -> ("States Out"=w589:string)  [unwired: 14 in]
      }
      frame "Metadata: Build Path" {
        n302 = Unbundle By Name(w647) -> ("Experiment.Instrument"=w644:T9, "Experiment.Device"=w643:string)
        n303 = Format Into String(w644) -> (resulting string=w636:string)  [unwired: 3 in, 1 out]
        n304 = xnode "Match Regular Expression"("input string"=w636, "regular expression"=" \\(") -> ("before match"=w634:string, "error out"=w633:errorcluster)  [unwired: 4 in, 3 out]
        n305 = call <vilib>:"Clear Errors.vi"("error in (no error)"=w633) -> ()  [unwired: 5 in, 2 out]
        n306 = Build Path(base path="Default Path", name or relative path=w634) -> (appended path=w645:path)
        n307 = Build Path(base path=w645, name or relative path=w643) -> (appended path=w642:path)
        n308 = call <userlib>:"MGI Create Directory Chain.vi"("Error In"=w641, "File Presence (Auto Detect)"=MGI_Create_Directory_Chain_Behavior_Enum."Path Does Not Contain a File", "Path"=w642) -> ("Error Out"=w640:errorcluster, "Duplicate Path"=w638:path)  [unwired: 7 in]
        "Device Folder" <- w638
        n309 = Bundle By Name(cluster=w647, "Experiment.Device Path"=w638) -> (w646:T24)
        n310 = call <vilib>:"Add State(s) to Queue__jki_lib_state_machine.vi"("State(s) in (\"\")"=w649) -> ("States Out"=w648:string)  [unwired: 14 in]
      }
      frame "Metadata: Update Control Experiment Wire" {
        # "IS Control Experiment Class wire"
        # "Not on Control Experiment Class wire"
        n311 = Unbundle By Name(w768) -> ("C.E."=w766:refnum<class "Control Experiment.lvclass">, "Experiment"=w770:T19, "Wiring Configuration"=w769:T21)
        n312 = Bundle By Name(cluster=w766, "Experiment"=w770, "Wiring Configuration"=w769) -> (w764:refnum<class "Control Experiment.lvclass">)
        n313 = Bundle By Name(cluster=w768, "C.E."=w764) -> (w767:T24)
        n314 = call <vilib>:"Add State(s) to Queue__jki_lib_state_machine.vi"("State(s) in (\"\")"=w772) -> ("States Out"=w771:string)  [unwired: 14 in]
      }
      frame "Metadata: Update Comments" {
        # "error 63 occurs when\nthe lockin isn't running\nI think we can clear here?"
        n315 = Unbundle By Name(w783) -> ("C.E."=w779:refnum<class "Control Experiment.lvclass">)
        n316 = call "Generate Comments.vi"("error in (no error)"=w774, "Control Experiment"=w779) -> ("error out"=w776:errorcluster, "Control Experiment out"=w778:refnum<class "Control Experiment.lvclass">)  [unwired: 6 in, 1 out]
        n317 = call <vilib>:"Clear Errors.vi"("error in (no error)"=w776, "specific error code to clear (0: all)"=63) -> ("error out"=w775:errorcluster)  [unwired: 4 in, 1 out]
        n318 = call "Read Comments.vi"("error in (no error)"=w775, "Control Experiment in"=w778) -> ("error out"=w773:errorcluster, "Comments"=→"Comments":string, "Control Experiment out"=w780:refnum<class "Control Experiment.lvclass">)  [unwired: 7 in]
        n319 = Bundle By Name(cluster=w783, "C.E."=w780) -> (w782:T24)
        n320 = call <vilib>:"Add State(s) to Queue__jki_lib_state_machine.vi"("State(s) in (\"\")"=w785) -> ("States Out"=w784:string)  [unwired: 14 in]
      }
      frame "Metadata: Write JSON" {
        w796 = T28 {"Device"={"Device"="", "User"="", "Time"="", "Computer Name"=""}, "Wiring"={"Lockin Ch"=[], "KH Electrodes"=[], "KH Labels"=[], "Other Electrodes"=[], "Other Labels"=[]}}  # Control Experiment JSON
        n321 = Unbundle By Name(w791) -> ("C.E."=w789:refnum<class "Control Experiment.lvclass">, "Experiment.Device"=w804:string, "Experiment.User"=w794:string)
        n322 = Unbundle By Name(w791) -> ("Lockin.AI"=w803:u32[], "Wiring Configuration.KH.Electrodes"=w802:string[], "Wiring Configuration.KH.Labels"=w801:string[], "Wiring Configuration.not KH.Electrodes"=w799:string[], "Wiring Configuration.not KH.Labels"=w798:string[])
        n323 = call "Get Date Time ISO.vi"() -> ("ISO 8601 date-time string"=w797:string)  [unwired: 9 in, 2 out]
        n324 = call "Get Computer Name.vi"() -> ("name"=w800:string)  [unwired: 10 in, 1 out]
        n325 = Bundle By Name(cluster=w796, "Device.Device"=w804, "Device.User"=w794, "Device.Time"=w797, "Device.Computer Name"=w800) -> (w795:T28)
        n326 = Bundle By Name(cluster=w795, "Wiring.Lockin Ch"=w803, "Wiring.KH Electrodes"=w802, "Wiring.KH Labels"=w801, "Wiring.Other Electrodes"=w799, "Wiring.Other Labels"=w798) -> (w790:T28)
        n327 = call "To JSON Text.vim"("error in (no error)"=w793, "Anything"=w790) -> ("error out"=w787:errorcluster, "<JSON>"=w786:string)  [unwired: 8 in]
        "JSON String" <- w786
        n328 = Bundle By Name(cluster=w789, "json"=w786) -> (w788:refnum<class "Control Experiment.lvclass">)
        n329 = Bundle By Name(cluster=w791, "C.E."=w788) -> (w792:T24)
        n330 = call <vilib>:"Add State(s) to Queue__jki_lib_state_machine.vi"("State(s) in (\"\")"=w806) -> ("States Out"=w805:string)  [unwired: 14 in]
      }
      frame "Metadata: Write FGV" {
        n331 = Unbundle By Name(w811) -> ("C.E."=w809:refnum<class "Control Experiment.lvclass">)
        n332 = call "Control Experiment FGV.vi"("Function"=enum16{"read", "write"}."write", "error in (no error)"=w807, "Control Experiment.lvclass"=w809) -> ("error out"=w808:errorcluster)  [unwired: 7 in, 1 out]
        n333 = call <vilib>:"Add State(s) to Queue__jki_lib_state_machine.vi"("State(s) in (\"\")"=w813) -> ("States Out"=w812:string)  [unwired: 14 in]
      }
      frame "Metadata: Read FGV" {
        n334 = call "Control Experiment FGV.vi"("Function"=enum16{"read", "write"}."read", "error in (no error)"=w817) -> ("error out"=w818:errorcluster, "Control Experiment.lvclass out"=w816:refnum<class "Control Experiment.lvclass">)  [unwired: 8 in]
        n335 = Bundle By Name(cluster=w814, "C.E."=w816) -> (w815:T24)
        n336 = call <vilib>:"Add State(s) to Queue__jki_lib_state_machine.vi"("State(s) in (\"\")"=w821) -> ("States Out"=w820:string)  [unwired: 14 in]
      }
      frame "---------- KH ----------" {
        n337 = call <vilib>:"Add State(s) to Queue__jki_lib_state_machine.vi"("State(s) in (\"\")"=w825) -> ("States Out"=w824:string)  [unwired: 14 in]
      }
      frame "KH: set KH 0" {
        # "initialize the Channel Settings array"
        # "remove duplicates"
        n338 = local read "KH Addresses"() -> (w828:refnum<visa-resource-name>[])
        n339 = call "Remove Duplicates From 1D Array.vim"("array"=w828) -> ("array with duplicates removed"=w827:refnum<visa-resource-name>[])  [unwired: 10 in]
        n340 = local write "KH Addresses"(w827) -> ()
        n341 = Initialize Array(T15 {"Channel"=enum."Channel 1", "Gain"=enum."10x", "Bandwidth Filter"=enum."ON", "Shunt Resistor"=enum."50 Ohms", "Coupling"=enum."DC", "Input Config"=enum."Differential"} ("Channel Settings"), 8 ("dimension size")) -> (w834:T15[])
        n342 = Empty Array?(array=w827) -> (empty?=w829:bool)
        n343 = case shown="True" w829 {
          tunnel: w826 -> [w846 w861]
          tunnel: [w845 w861] -> w832
          tunnel: [w844 string[] []] -> w830
          tunnel: w827 -> [w843 _]
          frame False {
            n344 = for {
              tunnel: w843 -> [_] mode=indexing
              tunnel: [w850] -> w844 mode=concatenating
              tunnel: w846 -> [w849]
              tunnel: [w848] -> w845
              i -> [w852]
              n345 = call "Number to Letter.vi"("Number"=w852) -> ("Letter"=w851:string)
              n346 = for {
                N: 8 -> [_]
                tunnel: w851 -> [w857]
                tunnel: [w856] -> w850 mode=indexing
                tunnel: w849 -> [w855]
                tunnel: [w854] -> w848
                i -> [w859]
                n347 = Increment(x=w859) -> (x+1=w853:i32)
                n348 = Format Into String(format string="%s %d", error in=w855, w857, w853) -> (resulting string=w856:string, error out=w854:errorcluster)  [unwired: 1 in]
              }
            }
          }
          frame True {
          }
        }
        n349 = Array Size(array=w827) -> (size(s)=w837:i32)
        n350 = Bundle(w834) -> (w833:cluster{T15[]})  [unwired: 1 in]
        n351 = Initialize Array(w833, w837) -> (w838:cluster{T15[]}[])
        n352 = Bundle By Name(cluster=w840, "Channel Settings"=w838) -> (w839:T24)
        n353 = property on="Ring" class="Ring (strict)"(error in=w832, "Strings []"=w830) -> (error out=w831:errorcluster)  [unwired: 1 in, 1 out]
        n354 = call <vilib>:"Add State(s) to Queue__jki_lib_state_machine.vi"("State(s) in (\"\")"=w842) -> ("States Out"=w841:string)  [unwired: 14 in]
      }
      frame "KH: set KH 1" {
        n355 = Unbundle By Name(w873) -> ("Channel Settings"=w862:cluster{"Channel Setting":T22}[], "KH.KH #"=w875:u16[], "KH.KH Gain"=w878:T3[], "Lockin.Electrode Config"=w876:T6[], "KH.KH Shunt Resistor"=w877:T4[], "KH All Buttons"=w874:T8)
        n356 = local read "Bandwidth Filter"() -> (w863:bool)
        n357 = local read "DC Coupled"() -> (w864:bool)
        n358 = for {
          tunnel: w876 -> [w903] mode=indexing
          tunnel: w878 -> [w902] mode=indexing
          tunnel: w877 -> [w901] mode=indexing
          tunnel: w875 -> [w897] mode=indexing
          tunnel: [w906] -> w869 mode=indexing
          tunnel: w874 -> [w905]
          tunnel: [w904] -> w867 mode=indexing
          tunnel: [w900] -> w868 mode=indexing
          shift-right: [w893] -> w871
          shift-left: w862 -> [w894]
          tunnel: w864 -> [w889]
          tunnel: w863 -> [w884]
          n359 = property on="Ring" class="Ring (strict)"() -> ("Strings []"=w899:string[])  [unwired: 2 in, 2 out]
          n360 = case shown="\"All Differential\"" w905 {
            tunnel: w903 -> [w925 _ _]
            tunnel: [w930 Input_Configuration-Enum."Ground" ("Input Config") Input_Configuration-Enum."Differential" ("Input Config")] -> w900
            tunnel: w902 -> [w929 w948 w951]
            tunnel: [w928 w948 w951] -> w904
            tunnel: w901 -> [w927 _ _]
            tunnel: [w926 Shunt-Enum."Open" ("Shunt Resistor") w949] -> w906
            frame "No Selection", Default {
              n361 = case shown="\"Current\"" w925 {
                tunnel: [Input_Configuration-Enum."Ground" ("Input Config") Input_Configuration-Enum."Differential" ("Input Config") Input_Configuration-Enum."SE+ (-gnd)" ("Input Config") Input_Configuration-Enum."Differential" ("Input Config") Input_Configuration-Enum."Differential" ("Input Config")] -> w930
                tunnel: [Shunt-Enum."Open" ("Shunt Resistor") w934 Shunt-Enum."Open" ("Shunt Resistor") Shunt-Enum."Open" ("Shunt Resistor") Shunt-Enum."50k Ohms" ("Shunt Resistor")] -> w926
                tunnel: w929 -> [w931 w935 w938 w942 w944]
                tunnel: [w931 w935 w938 w942 w944] -> w928
                tunnel: w927 -> [_ w934 _ _ _]
                frame "Ground", Default {
                }
                frame "Current" {
                }
                frame "Voltage (SE)" {
                }
                frame "Voltage (Diff)" {
                }
                frame "Gate" {
                }
              }
            }
            frame "All Ground" {
            }
            frame "All Differential" {
              n362 = local read "Defualt Shunt Resistor"() -> (w949:T4)
            }
          }
          n363 = To Long Integer(number=w897) -> (32bit integer=w898:i32)
          n364 = Index Array(array=w899, index=w898) -> (element=w896:string)
          n365 = Select(t=Coupling-Enum."DC" ("Coupling"), s=w889, f=Coupling-Enum."AC" ("Coupling")) -> (s? t:f=w886:T18)
          n366 = Scan From String(format string="%s %d", input string=w896) -> (error out=w890:errorcluster, output 1=w892:string, output 2=w891:i32)  [unwired: 4 in, 2 out]
          n367 = Select(t=Filter-Enum."ON" ("Bandwidth Filter"), s=w884, f=Filter-Enum."OFF" ("Bandwidth Filter")) -> (s? t:f=w882:T17)
          n368 = case shown="No Error" w890 {
            tunnel: w906 -> [w923 _]
            tunnel: w904 -> [w922 _]
            tunnel: w900 -> [w921 _]
            tunnel: w894 -> [w913 w924]
            tunnel: [w912 w924] -> w893
            tunnel: w892 -> [w911 _]
            tunnel: w891 -> [w910 _]
            tunnel: w886 -> [w908 _]
            tunnel: w882 -> [w907 _]
            frame No Error {
              n369 = Decrement(x=w910) -> (x-1=w909:i32)
              n370 = call "Letter to Number.vi"("Letter"=w911) -> ("Number"=w914:i32)
              n371 = Index Array(array=w913, index=w914) -> (element=w919:cluster{"Channel Setting":T22})
              n372 = Unbundle(w919) -> ("Channel Setting"=w918:T22)
              n373 = Index Array(array=w918, index=w909) -> (element=w917:T15)
              n374 = Bundle By Name(cluster=w917, "Channel"=w909, "Gain"=w922, "Input Config"=w921, "Shunt Resistor"=w923, "Coupling"=w908, "Bandwidth Filter"=w907) -> (w916:T15)
              n375 = Replace Array Subset(array=w918, new element=w916, index=w909) -> (w920:T22)
              n376 = Bundle("Channel Setting"=w920) -> (w915:cluster{"Channel Setting":T22})  [unwired: 1 in]
              n377 = Replace Array Subset(array=w913, new element=w915, index=w914) -> (w912:cluster{"Channel Setting":T22}[])
            }
            frame Error {
            }
          }
        }
        n378 = local write "KH All Buttons"(T8."No Selection" ("KH All Buttons")) -> ()
        n379 = Bundle By Name(cluster=w873, "Channel Settings"=w871, "KH.KH Gain"=w867, "KH.KH Configuration"=w868, "KH.KH Shunt Resistor"=w869) -> (w879:T24)
        n380 = local read "KH"() -> (w870:T5)
        n381 = Bundle By Name(cluster=w870, "KH Gain"=w867, "KH Configuration"=w868, "KH Shunt Resistor"=w869) -> (w866:T5)
        n382 = local write "KH"(w866) -> ()
        n383 = call <vilib>:"Add State(s) to Queue__jki_lib_state_machine.vi"("State(s) in (\"\")"=w881) -> ("States Out"=w880:string)  [unwired: 14 in]
      }
      frame "KH: set KH 2" {
        n384 = Unbundle By Name(w961) -> ("Channel Settings"=w964:cluster{"Channel Setting":T22}[])
        n385 = Unbundle By Name(w961) -> ("C.E."=w959:refnum<class "Control Experiment.lvclass">)
        n386 = Unbundle By Name(w959) -> ("KH7008"=w958:refnum<class "Instrument.KH7008.lvclass">[])
        n387 = for {
          tunnel: w957 -> [w979]
          tunnel: [w971] -> w952
          tunnel: w964 -> [w978] mode=indexing
          tunnel: w958 -> [w977] mode=indexing
          tunnel: [w970] -> w962 mode=concatenating
          tunnel: [w969] -> w956 mode=indexing
          n388 = Unbundle(w978) -> ("Channel Setting"=w974:T22)
          n389 = call <userlib>:"Write Channel Setting.vi"("error in (no error)"=w979, "Channel Setting"=w974, "KH7008 in"=w977) -> ("error out"=w975:errorcluster, "KH7008 out"=w976:refnum<class "Instrument.KH7008.lvclass">)  [unwired: 7 in]
          n390 = call <userlib>:"KH Control.vi"("error in"=w975, "KH7008"=w976) -> ("error out"=w973:errorcluster, "KH7008.lvclass out"=w972:refnum<class "Instrument.KH7008.lvclass">)  [unwired: 8 in]
          n391 = call <userlib>:"Read Gain.vi"("error in (no error)"=w973, "KH7008 in"=w972) -> ("error out"=w971:errorcluster, "Gain"=w970:dbl[], "KH7008 out"=w969:refnum<class "Instrument.KH7008.lvclass">)  [unwired: 7 in]
        }
        n392 = local read "Gain"() -> (w963:dbl[])
        n393 = Bundle By Name(cluster=w959, "KH7008"=w956) -> (w960:refnum<class "Control Experiment.lvclass">)
        n394 = call "Multiply Gains.vi"("Other Gain"=w963, "Gain"=w962) -> ("Gain x Other Gain"=w954:dbl[])
        n395 = Unbundle By Name(w960) -> ("Lockin"=w955:refnum<class "Instrument.Lockin.lvclass">)
        n396 = call <userlib>:"setInputGain.vi"("error in (no error)"=w952, "InputGain"=w954, "Instrument.Lockin in"=w955) -> ("error out"=w953:errorcluster)  [unwired: 7 in, 1 out]
        n397 = Bundle By Name(cluster=w961, "C.E."=w960) -> (w966:T24)
        n398 = call <vilib>:"Clear Errors.vi"("error in (no error)"=w953) -> ("error out"=w965:errorcluster)  [unwired: 5 in, 1 out]
        n399 = call <vilib>:"Add State(s) to Queue__jki_lib_state_machine.vi"("State(s) in (\"\")"=w968) -> ("States Out"=w967:string)  [unwired: 14 in]
      }
      frame "---------- Instruments ----------" {
        n400 = call <vilib>:"Add State(s) to Queue__jki_lib_state_machine.vi"("State(s) in (\"\")"=w983) -> ("States Out"=w982:string)  [unwired: 14 in]
      }
      frame "Instruments: Load Classes" {
        n401 = Unbundle By Name(w991) -> ("C.E."=w989:refnum<class "Control Experiment.lvclass">)
        n402 = disable-structure shown="Enabled" {
          disable-tunnel: w989 -> [w999 w1003]
          disable-tunnel: [w998 w1002] -> w986
          disable-tunnel: [w997 w1000] -> w988
          disable-tunnel: w987 -> [w996 w1001]
          frame Disabled {
            n403 = call "Load Instrument Classes.vi"("error in (no error)"=w996, "Control Experiment.lvclass"=w999) -> ("error out"=w997:errorcluster, "Control Experiment out"=w998:refnum<class "Control Experiment.lvclass">)  [unwired: 8 in]
          }
          frame Enabled {
            n404 = call "Load Instrument Classes_New.vi"("error in (no error)"=w1001, "C.E."=w1003) -> ("error out"=w1000:errorcluster, "Control Experiment"=w1002:refnum<class "Control Experiment.lvclass">)  [unwired: 8 in]
          }
        }
        n405 = Unbundle By Name(w986) -> ("KH7008"=w984:refnum<class "Instrument.KH7008.lvclass">[])
        n406 = for {
          tunnel: [w994] -> w985 mode=indexing
          tunnel: w984 -> [_] mode=indexing
          i -> [w995]
          n407 = Number To Decimal String(number=w995) -> (decimal integer string=w994:string)  [unwired: 1 in]
        }
        n408 = Bundle By Name(cluster=w991, "C.E."=w986) -> (w990:T24)
        n409 = property on="KH Addresses" class="Arr (strict)"("Val(Sgnl)"=w985) -> ()  [unwired: 2 in, 2 out]
        n410 = call <vilib>:"Add State(s) to Queue__jki_lib_state_machine.vi"("State(s) in (\"\")"=w993) -> ("States Out"=w992:string)  [unwired: 14 in]
      }
      frame "---------- Experiment VI ----------" {
        n411 = call <vilib>:"Add State(s) to Queue__jki_lib_state_machine.vi"("State(s) in (\"\")"=w1007) -> ("States Out"=w1006:string)  [unwired: 14 in]
      }
      frame "Experiment VI: Populate VI Ring" {
        n412 = call <userlib>:"Current VIs Parent Directory__ogtk.vi"() -> ("Parent Directory (+ Relative)"=w1024:path)  [unwired: 5 in]
        n413 = call <userlib>:"String to 1D Array__ogtk.vi"("delimiter (Tab)"="\n", "string"="----Sweep Control----\nSweep Control.vi\nContinuous B Sweep.vi") -> ("Array of Strings"=w1010:string[])  [unwired: 9 in]
        n414 = call <userlib>:"String to 1D Array__ogtk.vi"("delimiter (Tab)"="\n", "string"="----Transport----\nIV.vi\nIV_Sweep.vi\nLockin_time.vi\nLockin_Vsg.vi\nLockin_sweep.vi\nLockin_AIWFM_time.vi\nTHz_TimeDelay.vi\nSweep_AIWFM_time.vi") -> ("Array of Strings"=w1009:string[])  [unwired: 9 in]
        n415 = Strip Path(path=w1024) -> (stripped path=w1021:path)  [unwired: 1 out]
        n416 = Build Path(base path=w1021, name or relative path="SweepControl") -> (appended path=w1020:path)
        n417 = Build Path(base path=w1021, name or relative path="Transport") -> (appended path=w1016:path)
        n418 = for {
          tunnel: w1020 -> [w1034]
          tunnel: w1010 -> [w1033] mode=indexing
          tunnel: [w1032] -> w1013 mode=indexing
          n419 = Build Path(base path=w1034, name or relative path=w1033) -> (appended path=w1032:path)
        }
        n420 = for {
          tunnel: w1016 -> [w1031]
          tunnel: w1009 -> [w1030] mode=indexing
          tunnel: [w1029] -> w1012 mode=indexing
          n421 = Build Path(base path=w1031, name or relative path=w1030) -> (appended path=w1029:path)
        }
        n422 = Build Array (concatenate)(w1013, w1012) -> (w1011:path[])
        n423 = Build Array (concatenate)(w1010, w1009) -> (w1008:string[])
        n424 = Bundle By Name(cluster=w1015, "VI paths"=w1011) -> (w1014:T24)
        n425 = property on="Ring" class="Ring (strict)"("Strings []"=w1008) -> ()  [unwired: 2 in, 2 out]
        n426 = call <vilib>:"Add State(s) to Queue__jki_lib_state_machine.vi"("State(s) in (\"\")"=w1028) -> ("States Out"=w1027:string)  [unwired: 14 in]
      }
      frame "Experiment VI: Open VI" {
        n427 = Unbundle By Name(w1040) -> ("VI paths"=w1039:path[])
        n428 = Index Array(array=w1039, index="Ring") -> (element=w1037:path)
        n429 = call "Open Experiment VI.vi"("error in (no error)"=w1036, "Path"=w1037) -> ("error out"=w1035:errorcluster)  [unwired: 9 in]
        n430 = call <vilib>:"Add State(s) to Queue__jki_lib_state_machine.vi"("State(s) in (\"\")"=w1042) -> ("States Out"=w1041:string)  [unwired: 14 in]
      }
      frame "Experiment VI: Open Lockin" {
        n431 = call "Open Lockin.vi"("error in (no error)"=w1044) -> ("error out"=w1043:errorcluster)  [unwired: 10 in]
        n432 = call <vilib>:"Add State(s) to Queue__jki_lib_state_machine.vi"("State(s) in (\"\")"=w1047) -> ("States Out"=w1046:string)  [unwired: 14 in]
      }
      frame "---------- PGSQL ----------" {
        n433 = call <vilib>:"Add State(s) to Queue__jki_lib_state_machine.vi"("State(s) in (\"\")"=w1051) -> ("States Out"=w1050:string)  [unwired: 14 in]
      }
      frame "PGSQL: Start Logger" {
        n434 = Unbundle By Name(w1053) -> ("Logger"=w1058:refnum<class "Logger.PGSQL.lvclass">)
        n435 = call <vilib>:"Create.vi"("error in (no error)"=w1055, "SMO"=w1058) -> ("error out"=w1057:errorcluster, "SMO out"=w1059:refnum<class "Logger.PGSQL.lvclass">)  [unwired: 7 in, 1 out]
        n436 = call <vilib>:"Start.vi"("error in (no error)"=w1057, "SMO"=w1059) -> ("error out"=w1054:errorcluster, "SMO out"=w1056:refnum<class "Logger.PGSQL.lvclass">)  [unwired: 8 in]
        n437 = Bundle By Name(cluster=w1053, "Logger"=w1056) -> (w1052:T24)
        n438 = call <vilib>:"Add State(s) to Queue__jki_lib_state_machine.vi"("State(s) in (\"\")"=w1061) -> ("States Out"=w1060:string)  [unwired: 14 in]
      }
      frame "PGSQL: Write" {
        w1073 = "" ("f")
        n439 = Unbundle By Name(w1077) -> ("Logger"=w1071:refnum<class "Logger.PGSQL.lvclass">, "Experiment.Instrument"=w1062:T9, "Experiment.Device"=w1076:string, "Experiment.User"=w1075:string)
        n440 = local read "I'm Finished Taking Data!"() -> (w1074:bool)
        n441 = Not(x=w1074) -> (.not. x?=w1072:bool)
        n442 = call "Device and User PGSQL Paths.vi"("instrument"=w1062) -> ("User Path"=w1064:string, "Device Path"=w1070:string)  [unwired: 5 in]
        n443 = Select(t=w1076, s=w1072, f=w1073) -> (s? t:f=w1069:string)
        n444 = Select(t=w1075, s=w1072, f=w1073) -> (s? t:f=w1063:string)
        n445 = call <userlib>:"Logger.PGSQL.WriteVariable.vi"("error in (no error)"=w1067, "Data"=w1069, "Address"=w1070, "Logger"=w1071) -> ("error out"=w1066:errorcluster, "Logger out"=w1068:refnum<class "Logger.PGSQL.lvclass">)  [unwired: 6 in]
        n446 = call <userlib>:"Logger.PGSQL.WriteVariable.vi"("error in (no error)"=w1066, "Data"=w1063, "Address"=w1064, "Logger"=w1068) -> ("error out"=w1065:errorcluster)  [unwired: 6 in, 1 out]
        n447 = call <vilib>:"Add State(s) to Queue__jki_lib_state_machine.vi"("State(s) in (\"\")"=w1079) -> ("States Out"=w1078:string)  [unwired: 14 in]
      }
    }
  }
  "Error Out" <- w2
  n448 = Unbundle By Name(w6) -> ("C.E."=→"Control Experiment":refnum<class "Control Experiment.lvclass">)
